vi "pyonpyon3.6.vi"() -> ()   [LabVIEW 2013]
uses:
  impl/pp3_CTL_State.ctl
  impl/pp3_CTL_Trial.ctl
  labolabo2/waveforms/WFTypes.ctl
  impl/pp3_CTL_TrialType.ctl
  <vilib>/Utility/file.llb/Read From Spreadsheet File (string).vi
  labolabo2/array/impl/NullArray_I.vi
  labolabo2/array/impl/ArrayFirst_S.vi
  <vilib>/userdefined/High Color/IMAQdx.ctl
  impl/pp3_CTL_SessionInfo.ctl
  impl/pp3_CTL_StateInfo.ctl
  impl/pp3_CTL_SessionParamDynamic.ctl
  <vilib>/sound2/lvsound2.llb/Sound Output Task ID.ctl
  impl/pp3_CTL_SessionParam.ctl
  impl/pp3c_CTL_DaqStatusVariable.ctl
panel:
  out "Session List Valid":bool=TRUE
  in  "Refresh info":bool
  in  "Session List Hidden":u8[](array[numeric])=[1, 1, 1, 2, 1, 2, 2, 1, 1, 2, 1, 2, 2, 1, 2, 2, 2, 1, 2, 1, 2, 2, 1, 1, 2, 2, 2, 1, 2, 2, 2, 1, 1, 2, 1, 1, 1, 2, 1, 1, 2, 1, 2, 2, 1, 1, 1, 2, 1, 2, 2, 2, 1, 1, 2, 2, 2, 1, 1, 2, 2, 1, 2, 1, 2, 1, 1, 2, 1, 1, 2, 1, 2, 1, 1, 2, 1, 2, 1, 2, 1, 2, 1, 2, 1, 2, 1, 2, 2, 1] min=1 step=1
  out "concatenated string":string="OS Name:                   Microsoft Wi\rOS Version:                6.1.7601 Service Pack 1 Build 7601\rSystem Type:               x64-based PC\rTime Zone:                 (UTC+01:00) Amsterdam, Berli\rTotal Physical Memory:     7,657 MB"
  out "Info VI Revision":string="1300" caption="Rev #"
  out "Info Hostname":string="PCR6985-17"
  out "Session list display":string[][](table)=[["1", "1", "1", "2", "1"], ["2", "2", "1", "1", "2"], ["1", "2", "2", "1", "2"], ["2", "2", "1", "2", "1"], ["2", "2", "1", "1", "2"], ["2", "2", "1", "2", "2"], ["2", "1", "1", "2", "1"], ["1", "1", "2", "1", "1"], ["2", "1", "2", "2", "1"], ["1", "1", "2", "1", "2"], ["2", "2", "1", "1", "2"], ["2", "2", "1", "1", "2"], ["2", "1", "2", "1", "2"], ["1", "1", "2", "1", "1"], ["2", "1", "2", "1", "1"], ["2", "1", "2", "1", "2"], ["1", "2", "1", "2", "1"], ["2", "1", "2", "2", "1"]]
  in  "Trial Types Control":enum32{"Trial Types Control"}(tab)
  out "Trial Types File Path":path=path "E:/Data/SPP.Coulb1/trial types/01_02__FM2k4k_4k2k.pp2tt.tsv"
  in  "Save Trial Types":bool
  in  "Load Trial Types":bool
  out "Trial Types Valid":bool=TRUE
  in  "Trial Types":T1[](array[typedef])=[{"Trial Type Number"=191, "Trial Type"=enum."GO", "Trial Weight"=1, "Shock (mA)"=-1.0, "Duration (ms)"=250.0, "Sound Type"=enum."01 DC", "Stim P1"=1000.0, "Stim P2"=0.0, "Stim P3"=0.0, "Stim P4"=1001.0, "DAQ Amplitude (V)"=0.0}, {"Trial Type Number"=192, "Trial Type"=enum."GO", "Trial Weight"=1, "Shock (mA)"=-1.0, "Duration (ms)"=250.0, "Sound Type"=enum."01 DC", "Stim P1"=1000.0, "Stim P2"=0.0, "Stim P3"=0.0, "Stim P4"=1002.0, "DAQ Amplitude (V)"=0.0}, {"Trial Type Number"=193, "Trial Type"=enum."GO", "Trial Weight"=1, "Shock (mA)"=-1.0, "Duration (ms)"=250.0, "Sound Type"=enum."01 DC", "Stim P1"=1000.0, "Stim P2"=0.0, "Stim P3"=0.0, "Stim P4"=1003.0, "DAQ Amplitude (V)"=0.0}, {"Trial Type Number"=255, "Trial Type"=enum."NOGO", "Trial Weight"=3, "Shock (mA)"=-1.0, "Duration (ms)"=250.0, "Sound Type"=enum."01 DC", "Stim P1"=1000.0, "Stim P2"=0.0, "Stim P3"=0.0, "Stim P4"=0.0, "DAQ Amplitude (V)"=0.0}] {"DAQ Amplitude (V)" min=0.0 max=5.0 format="%_4g"; "Shock (mA)" min=-1.0 max=5.0; "Trial Weight" step=1; "Duration (ms)" min=0.0 max=1.0; "Trial Type Number" min=1 max=256 step=1}
  in  "Session List Control":enum32{"Session List Control"}(tab)
  out "Session List File Path":path
  in  "Load Session List":bool
  in  "Save Session List":bool
  in  "Generate Session List":bool
  in  "Total Trials":i32=90 min=3 max=122 step=1
  in  "Pseudo-Gell. Start":i32=2 min=0 max=3 step=1
  in  "60 trials":bool
  in  "90 trials":bool
  in  "test trials":bool
  in  "Daq config":T4={"Sound AO"="Dev6/ao0", "Shock intesity AO"="Dev6/ao1", "Code_LED DO"="Dev6/port1:2", "Switch DI"="Dev6/port0/line0", "Webcam"="cam9", "Sound AO task"="", "Sound card task"=0, "Shock intensity AO task"="", "Code_LED DO task"="", "Switch DI task"="", "AO <=> Sound card"=FALSE, "Sound card"=0, "sample rate"=100000.0, "Variable shock"=TRUE, "Webcam on"=TRUE, "Waveform memo"={"t0"=timestamp(0 s since 1904-01-01), "dt"=1.0, "Y"=[]}, "First time"=FALSE, "Tone trigger"="PFI1", "Master-9 DO"="Dev6/port0/line5:7", "Master-9 DO task"=""} {"sample rate" min=8000.0; "Sound card task" format="%.0x"}
  out "Image":T7(plugin-control)
  in  "Session param (dynamic)":T8={"Def M shock (uA)"=700.0, "Def F shock (uA)"=140.0}
  in  "stop":bool
  in  "Pause":bool
  out "State info":T9={"Curr  tr"=90, "Curr (ms)"=22027788, "Cum (ms)"=2126369, "Run loop diff"=12, "Tone countdown (ms)"=777777, "Countdown (ms)"=0, "Curr State"=enum."15 Done", "Prev State"=enum."14 Intertrial Interval", "Rw"=FALSE, "Sw"=TRUE, "Tone\nGate"=FALSE, "Punish"=FALSE, "Current DAQ DO Int"=0, "Current Loaded Trial"={"Trial Type Number"=1, "Trial Type"=enum."GO", "Trial Weight"=1, "Shock (mA)"=700.0, "Duration (ms)"=250.0, "Sound Type"=enum."04 FM Sweep", "Stim P1"=2000.0, "Stim P2"=4000.0, "Stim P3"=0.0, "Stim P4"=0.0, "DAQ Amplitude (V)"=1.0}, "Next Trial (for display purposes)"={"Trial Type Number"=1, "Trial Type"=enum."GO", "Trial Weight"=1, "Shock (mA)"=-1.0, "Duration (ms)"=250.0, "Sound Type"=enum."04 FM Sweep", "Stim P1"=2000.0, "Stim P2"=4000.0, "Stim P3"=0.0, "Stim P4"=0.0, "DAQ Amplitude (V)"=1.0}, "Total trials memo"=90, "State start cum memo (ms)"=2111369, "Last dur jump time memo (ms)"=0, "Last dur shock time memo (ms)"=6007, "Tone repeat memo (ms)"=0, "Webcam on"=FALSE, "Webcam recording"=FALSE, "State update flag"=FALSE, "Last loaded shock voltage"=0.35000000000000003, "Vid upd"=enum."6"} {"Current DAQ DO Int" format="%016b"; "Next Trial (for display purposes)"."DAQ Amplitude (V)" min=0.0 max=5.0 format="%_4g"; "Next Trial (for display purposes)"."Shock (mA)" min=-1.0 max=5.0; "Next Trial (for display purposes)"."Trial Weight" step=1; "Next Trial (for display purposes)"."Duration (ms)" min=0.0 max=1.0; "Next Trial (for display purposes)"."Trial Type Number" min=1 max=256 step=1; "Current Loaded Trial"."DAQ Amplitude (V)" min=0.0 max=5.0 format="%_4g"; "Current Loaded Trial"."Shock (mA)" min=-1.0 max=5.0; "Current Loaded Trial"."Trial Weight" step=1; "Current Loaded Trial"."Duration (ms)" min=0.0 max=1.0; "Current Loaded Trial"."Trial Type Number" min=1 max=256 step=1}
  in  "Session parameters":T11={"Log File Directory Root"=path "E:/Data/SPP.Coulb1", "Subject Name"="SPP074", "Tone repeat (ms)"=0, "Habit tr0 (s)"=180, "ITI min\n(s)"=6, "ITI max\n(s)"=16, "Stay \n(s)"=3, "Run"=TRUE, "Jump time\n(s)"=4, "Start trial"=0, "Log File Directory"=path "E:/Data/SPP.Coulb1/SPP074/161224/161555", "Shock \ndur (s)"=6, "Pre click \n(V)"=0.1, "Click\ndel (s)"=1.0, "Reward CR"=FALSE} {"Click\ndel (s)" min=0.0 step=1.0; "Pre click \n(V)" min=0.0 max=1.0 step=1.0; "Shock \ndur (s)" min=0 step=1; "Stay \n(s)" min=0 step=1; "Start trial" step=1; "Jump time\n(s)" min=0 step=1; "Tone repeat (ms)" min=0 max=1000 step=1; "ITI min\n(s)" min=0 step=1; "ITI max\n(s)" min=0 step=1; "Habit tr0 (s)" min=0 step=1}
  out "Runtime Errors":errorcluster
  in  "Refresh":bool
  out "Session info":T12={"Total  Tr"=90, "G Tr"=45, "G Jump"=0, "G Jump%"=0.0, "N Tr"=45, "N Jump"=1, "N Jump%"=2.2222222222222223, "T Tr"=0, "T Jump"=0, "T Jump%"=nan, "M shock dur (ms)"=6003.133333333333, "F shock dur (ms)"=6005.0, "H latency (ms)"=0.0, "F latency (ms)"=3939.0, "T jump latency (ms)"=0.0} {"T Jump%" format="%.3g"; "N Jump%" format="%.3g"; "G Jump%" format="%.3g"}
  # "Pyonpyon Labview  v3.5 \n(2017.3 KT -- opto trig A)"
  # "60 trials:  180-14-24-5\n90 trials:  180-6-16-3"
  # "Code"
  # "Type"
  # "P 1"
  # "P 2"
  # "P 3"
  # "P 4 (opto)"
  # "Weight"
  # "Shock"
  # "Dur (ms)"
  # "DAQ Ampl (V)"
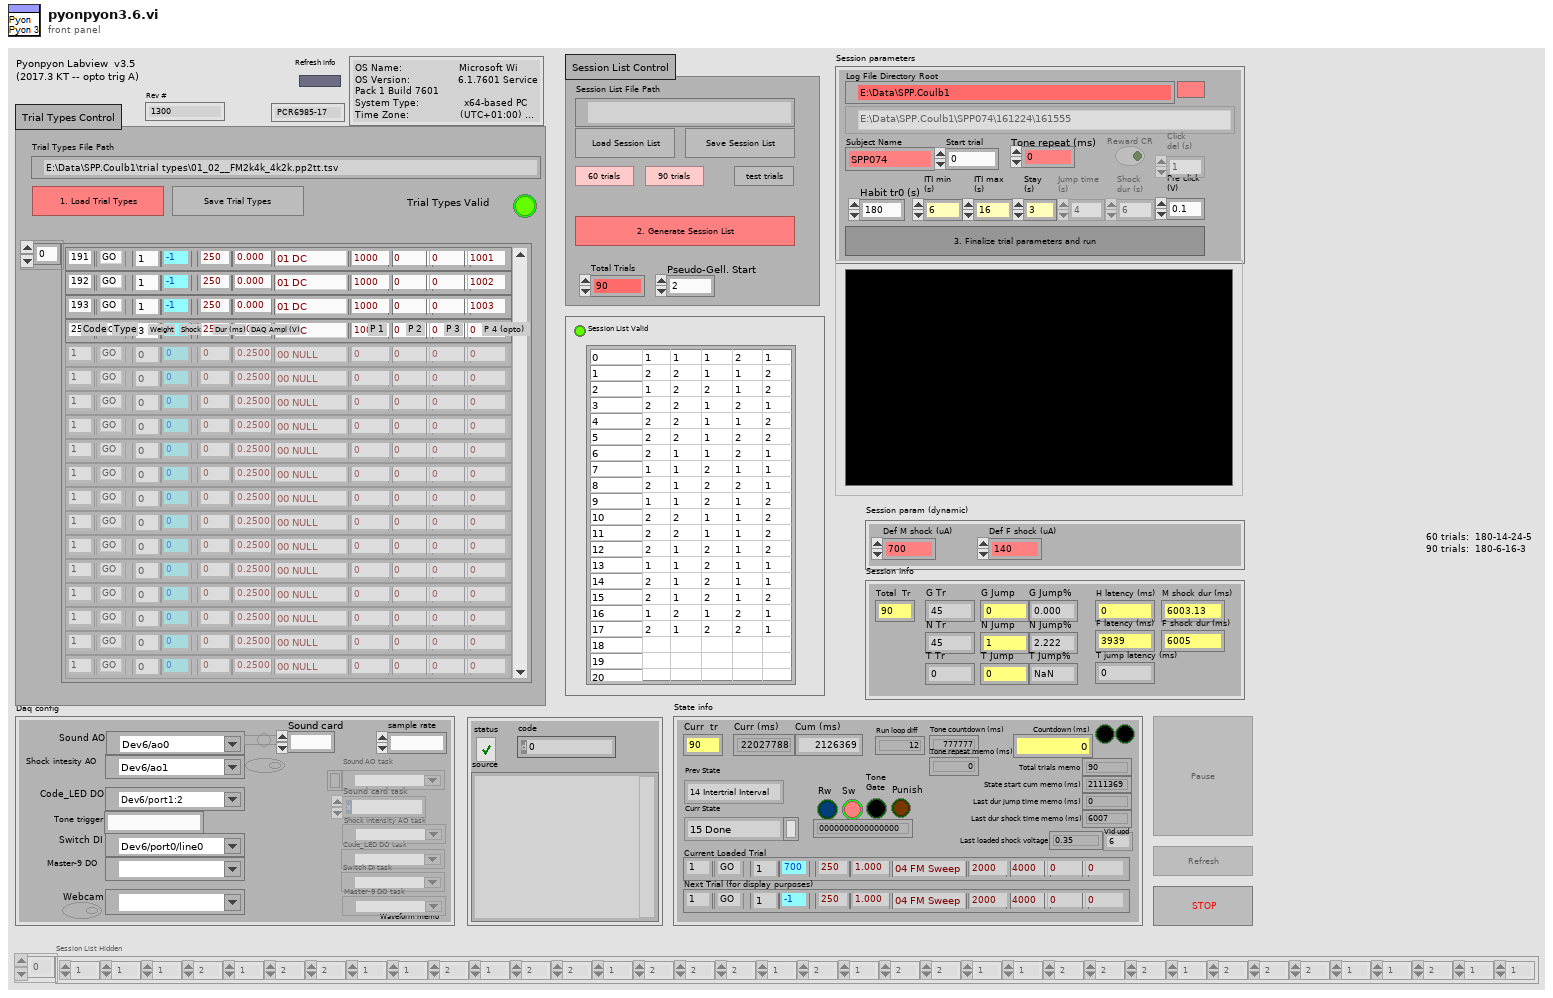
[diagram p1: front panel]
types:
  T1 = typedef "pp3_CTL_Trial.ctl" = cluster{"Trial Type Number":i16, "Trial Type":T2, "Trial Weight":u32, "Shock (mA)":dbl, "Duration (ms)":dbl, "Sound Type":T3, "Stim P1":dbl, "Stim P2":dbl, "Stim P3":dbl, "Stim P4":dbl, "DAQ Amplitude (V)":dbl}
  T2 = typedef "pp3_CTL_TrialType.ctl" = enum16{"OFF", "GO", "NOGO", "TEST"}
  T3 = typedef "WFTypes.ctl" = enum16{"00 NULL", "01 DC", "02 Noise", "03 Pure Tone", "04 FM Sweep"}
  T4 = typedef "pp3c_CTL_DaqStatusVariable.ctl" = cluster{"Sound AO":tag, "Shock intesity AO":tag, "Code_LED DO":tag, "Switch DI":tag, "Webcam":T5, "Sound AO task":refnum<k21>, "Sound card task":T6, "Shock intensity AO task":refnum<k21>, "Code_LED DO task":refnum<k21>, "Switch DI task":refnum<k21>, "AO <=> Sound card":bool, "Sound card":u32, "sample rate":dbl, "Variable shock":bool, "Webcam on":bool, "Waveform memo":waveform(dbl), "First time":bool, "Tone trigger":string, "Master-9 DO":tag, "Master-9 DO task":refnum<k21>}
  T5 = typedef "IMAQdx.ctl" = refnum<k21>
  T6 = typedef "Sound Output Task ID.ctl" = u32
  T7 = typedef "IMAQ Image.ctl" = refnum<image>
  T8 = typedef "pp3_CTL_SessionParamDynamic.ctl" = cluster{"Def M shock (uA)":dbl, "Def F shock (uA)":dbl}
  T9 = typedef "pp3_CTL_StateInfo.ctl" = cluster{"Curr  tr":u16, "Curr (ms)":u32, "Cum (ms)":i64, "Run loop diff":i64, "Tone countdown (ms)":i64, "Countdown (ms)":i64, "Curr State":T10, "Prev State":T10, "Rw":bool, "Sw":bool, "Tone\nGate":bool, "Punish":bool, "Current DAQ DO Int":u16, "Current Loaded Trial":T1, "Next Trial (for display purposes)":T1, "Total trials memo":i64, "State start cum memo (ms)":i64, "Last dur jump time memo (ms)":i64, "Last dur shock time memo (ms)":i64, "Tone repeat memo (ms)":i64, "Webcam on":bool, "Webcam recording":bool, "State update flag":bool, "Last loaded shock voltage":dbl, "Vid upd":enum16{"0", "1", "2", "3", "4", "5", "6", "7", "8", "9"}}
  T10 = typedef "pp3_CTL_State.ctl" = enum8{"0 NULL", "1 Habituation", "2 (Load Trial)", "3 Stay Period", "4 Load Audio/Click Delay", "5 GO Trial", "6 GO Jumped", "7 GO Timeout", "8 NOGO Trial", "9 NOGO Jumped", "10 NOGO Timeout", "11 TEST Trial", "12 TEST Jumped", "13 TEST Timeout", "14 Intertrial Interval", "15 Done"}
  T11 = typedef "pp3_CTL_SessionParam.ctl" = cluster{"Log File Directory Root":path, "Subject Name":string, "Tone repeat (ms)":i32, "Habit tr0 (s)":i32, "ITI min\n(s)":i32, "ITI max\n(s)":i32, "Stay \n(s)":i32, "Run":bool, "Jump time\n(s)":i32, "Start trial":u16, "Log File Directory":path, "Shock \ndur (s)":i32, "Pre click \n(V)":dbl, "Click\ndel (s)":dbl, "Reward CR":bool}
  T12 = typedef "pp3_CTL_SessionInfo.ctl" = cluster{"Total  Tr":u32, "G Tr":u32, "G Jump":u32, "G Jump%":dbl, "N Tr":u32, "N Jump":u32, "N Jump%":dbl, "T Tr":u32, "T Jump":u32, "T Jump%":dbl, "M shock dur (ms)":dbl, "F shock dur (ms)":dbl, "H latency (ms)":dbl, "F latency (ms)":dbl, "T jump latency (ms)":dbl}
  T13 = enum8{"Enabled", "Disabled", "Disabled and Grayed Out"}
  T14 = enum16{"open", "replace", "create", "open or create", "replace or create", "replace or create with confirmation"}
  T15 = typedef "imagedata.ctl" = cluster{"image type":i32, "image depth":i32, "image":u8[], "mask":u8[], "colors":u32[], "Rectangle":cluster{"left":i16, "top":i16, "right":i16, "bottom":i16}}
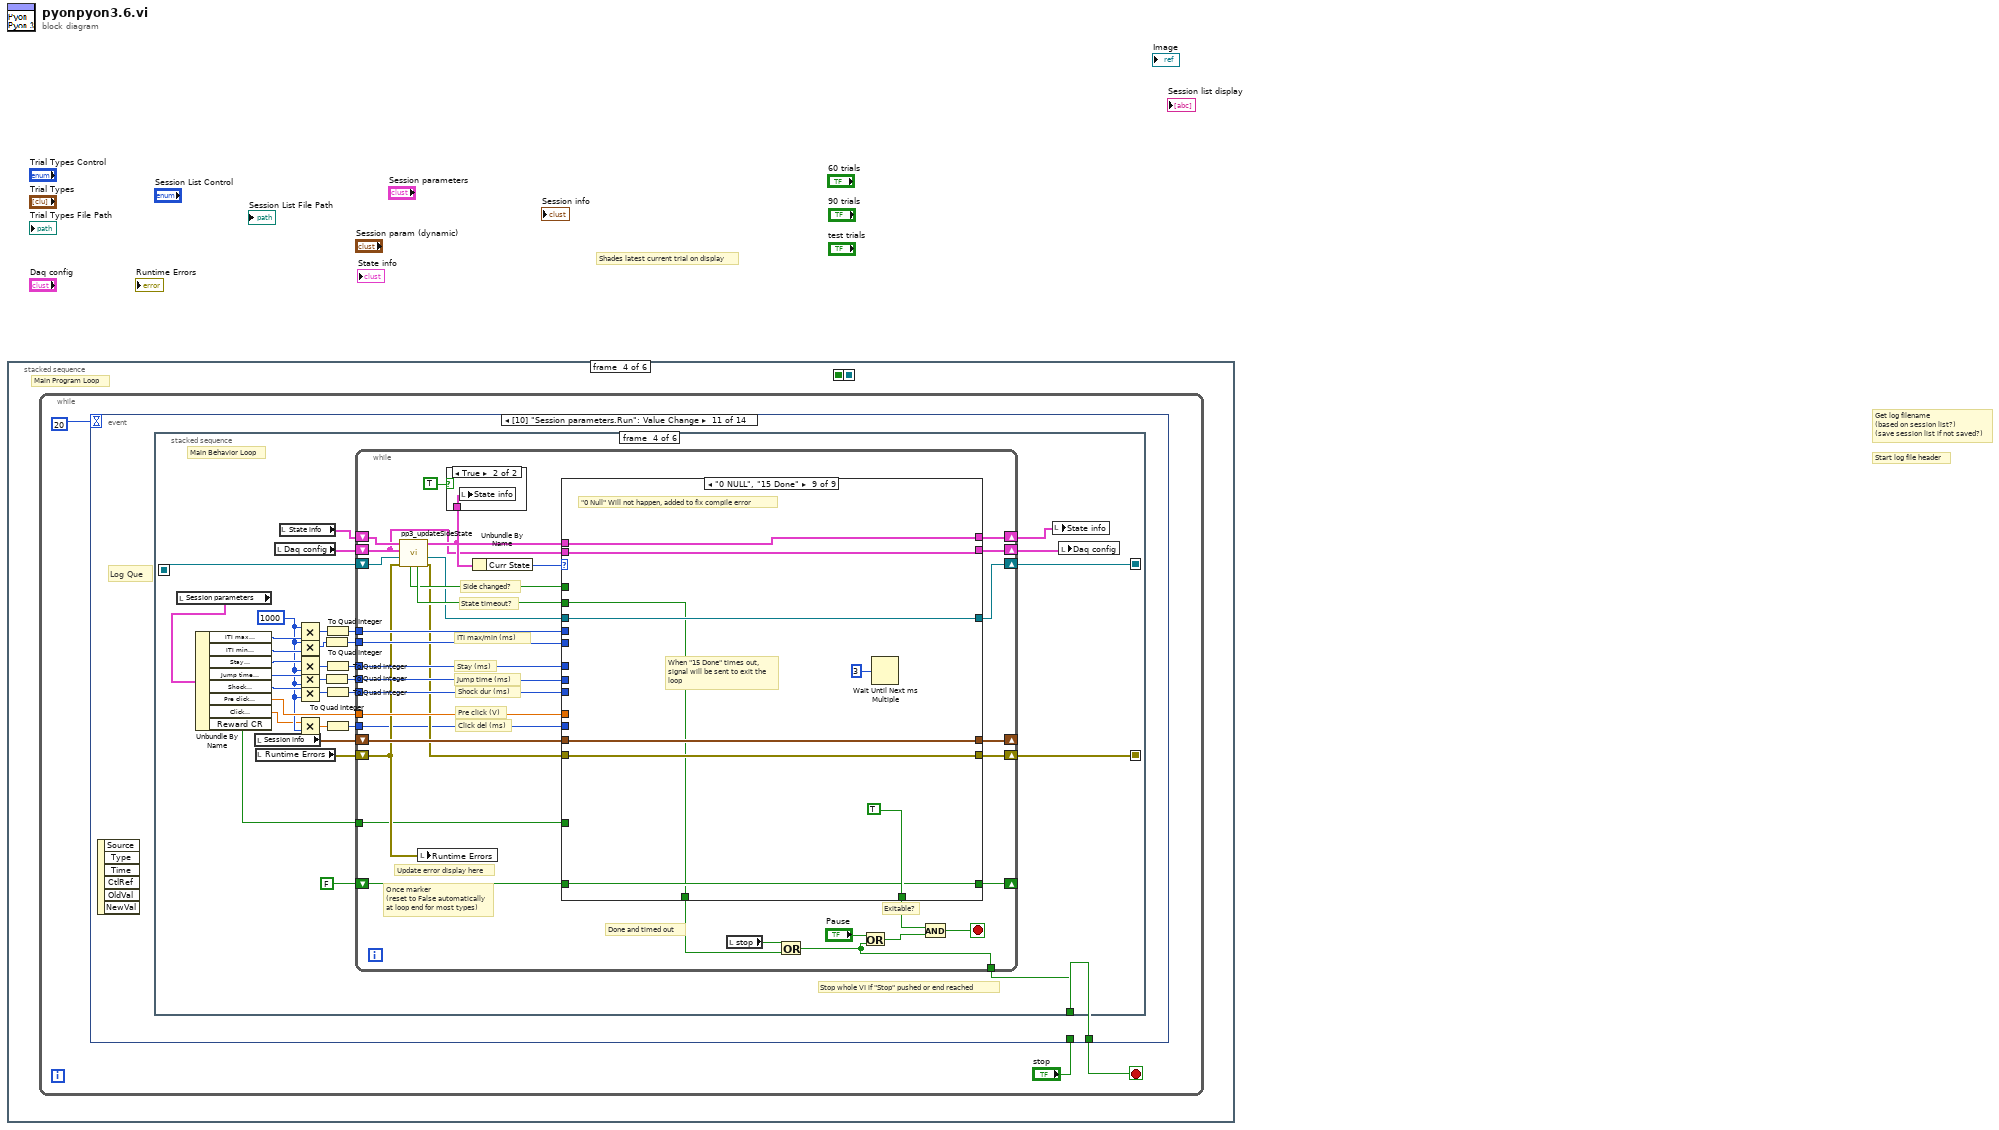
[diagram p0: block diagram]
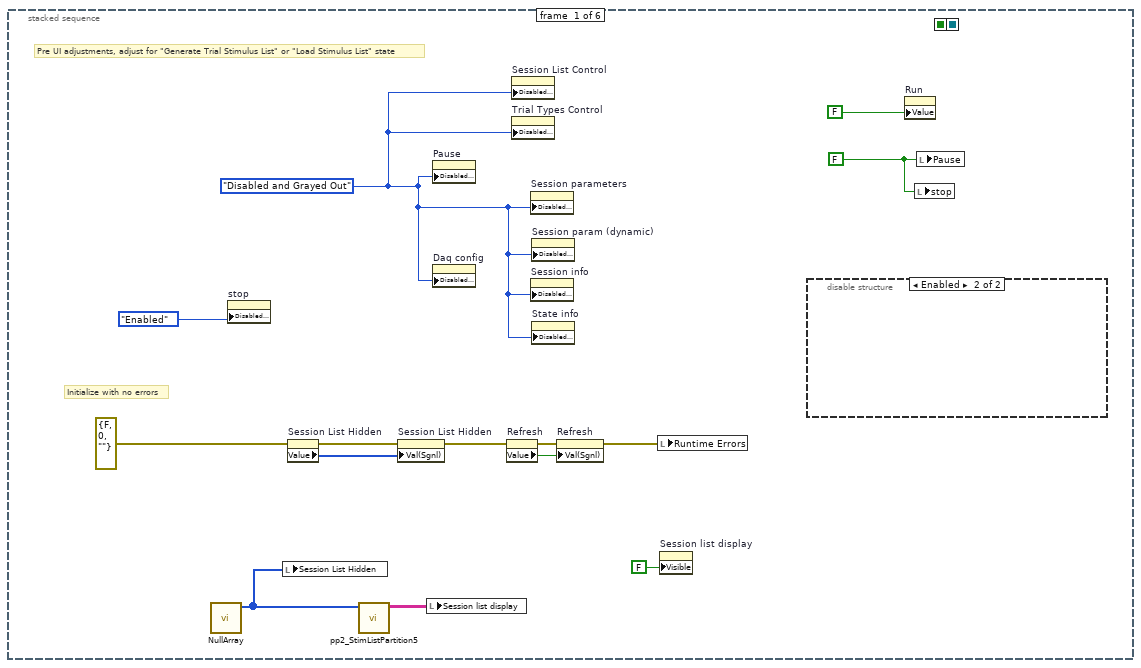
[diagram p2: hidden frame]
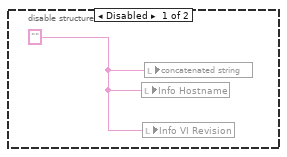
[diagram p3: hidden frame]
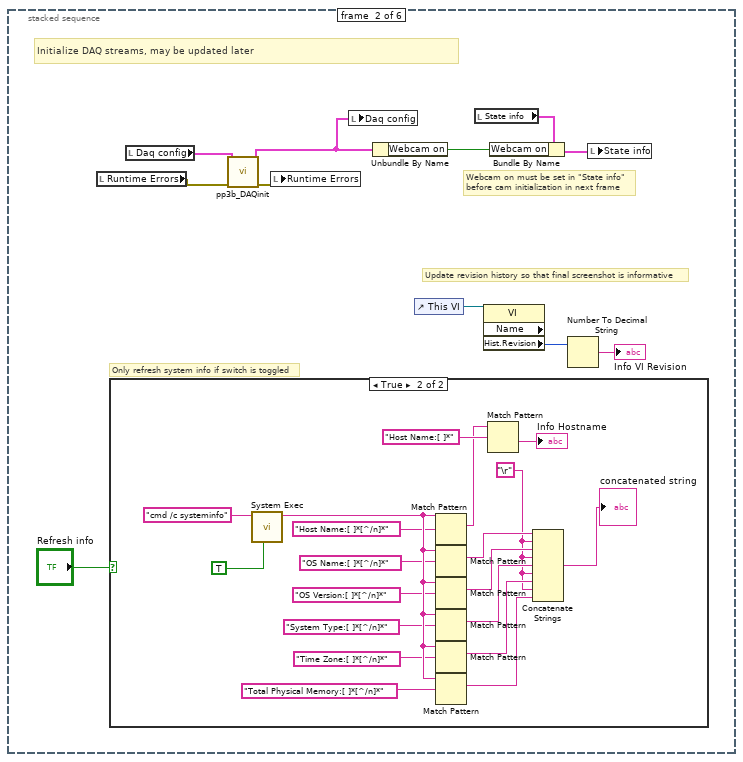
[diagram p4: hidden frame]
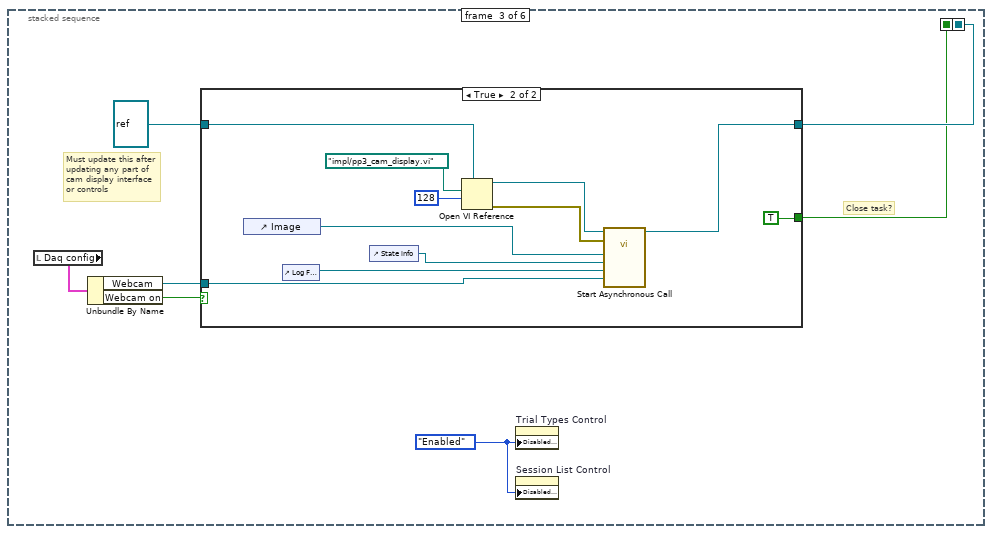
[diagram p6: hidden frame]
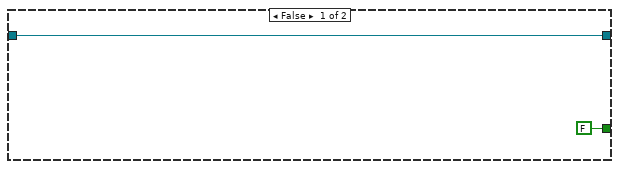
[diagram p7: hidden frame]
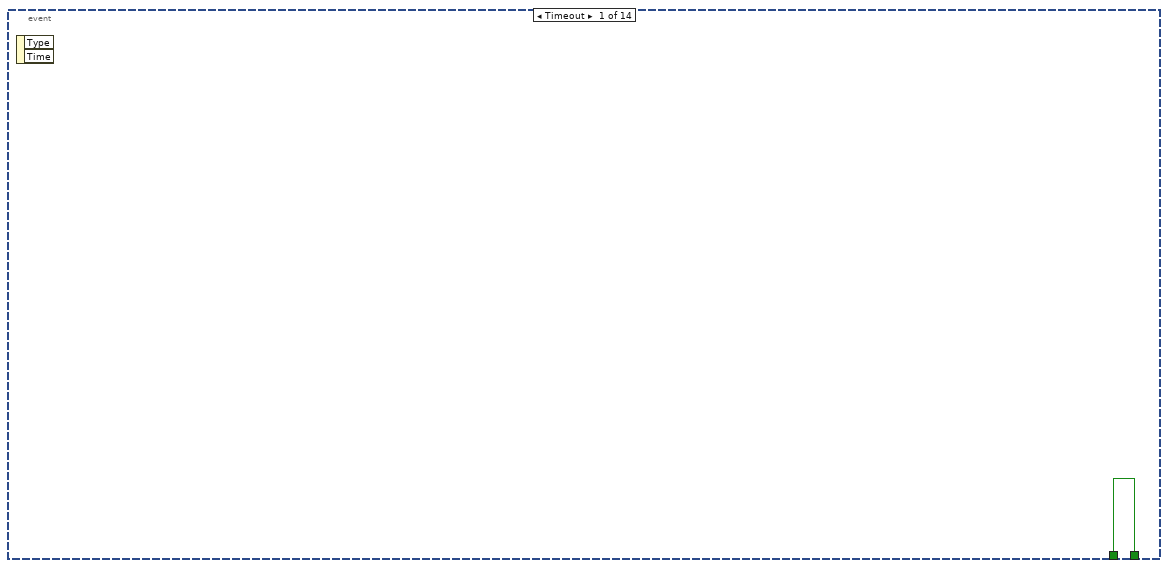
[diagram p8: hidden frame]
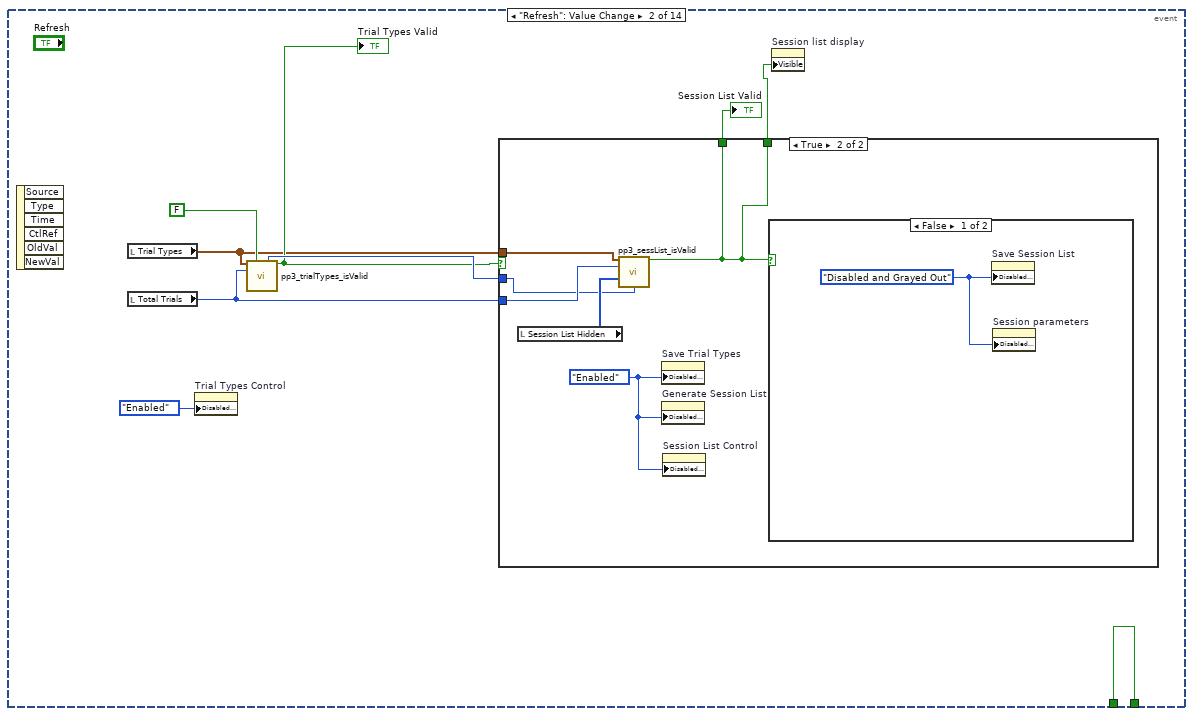
[diagram p9: hidden frame]
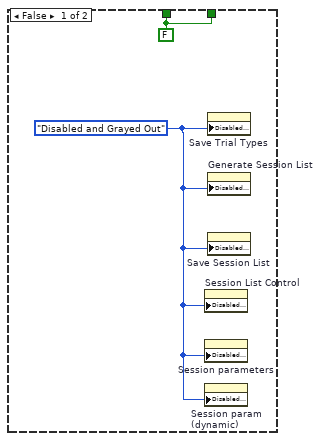
[diagram p10: hidden frame]
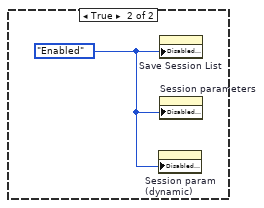
[diagram p11: hidden frame]
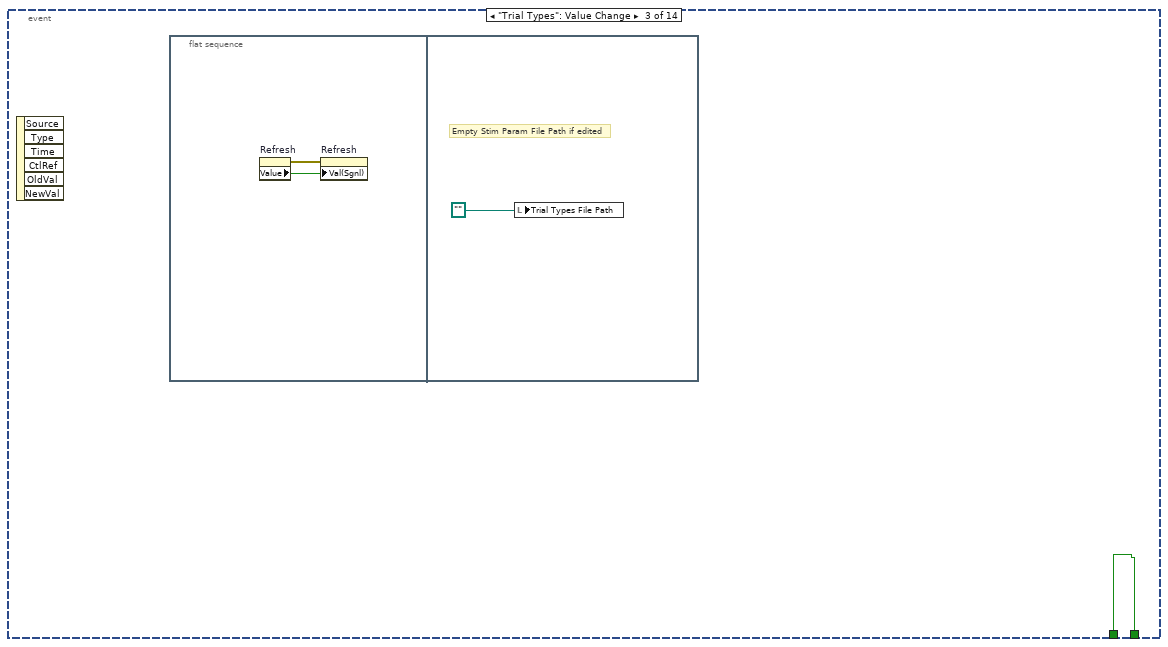
[diagram p12: hidden frame]
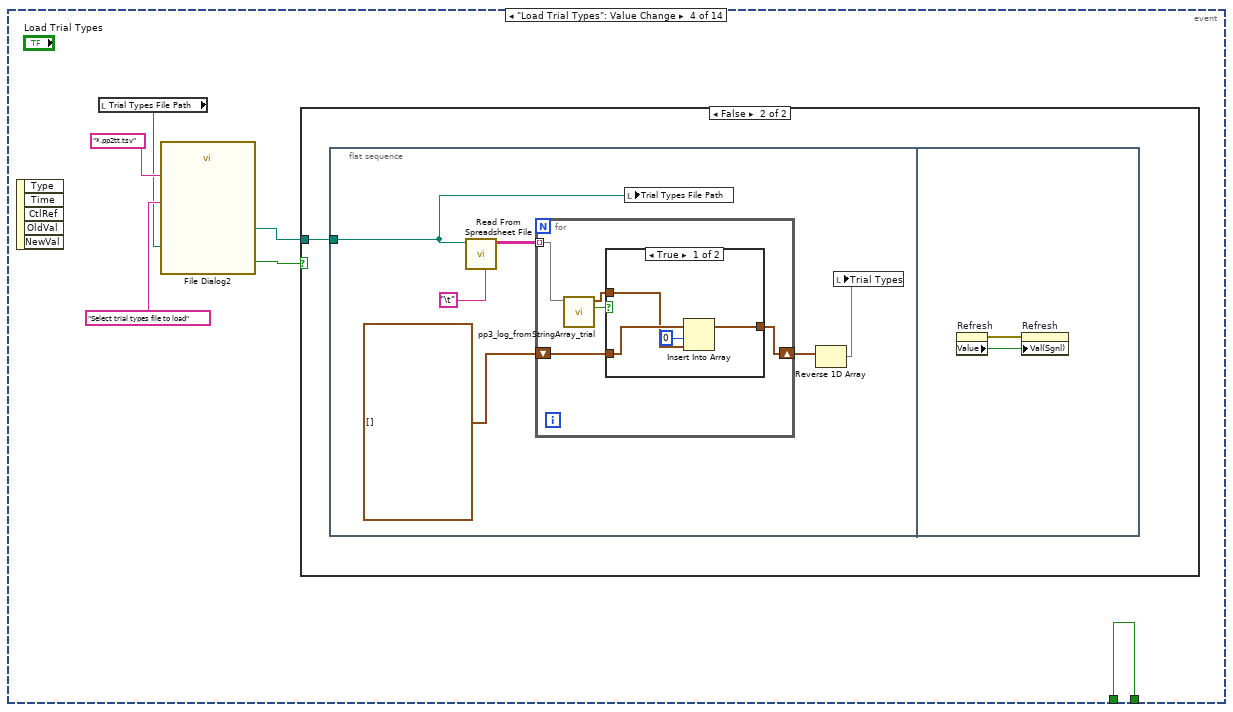
[diagram p13: hidden frame]
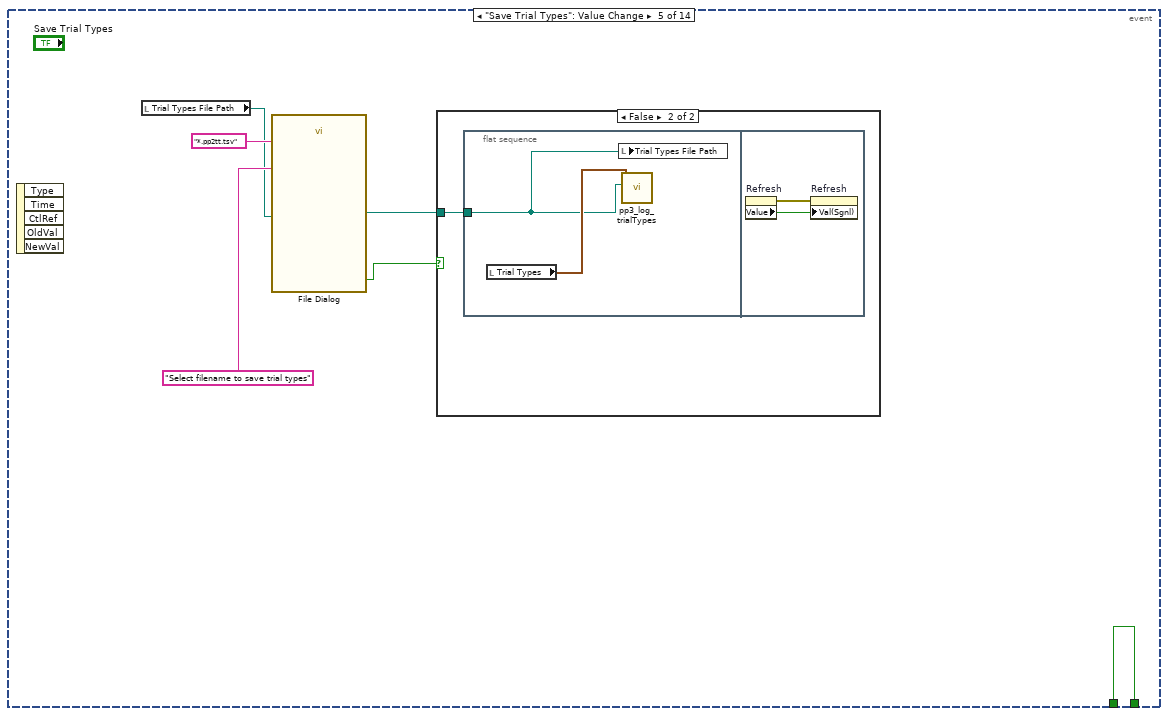
[diagram p16: hidden frame]
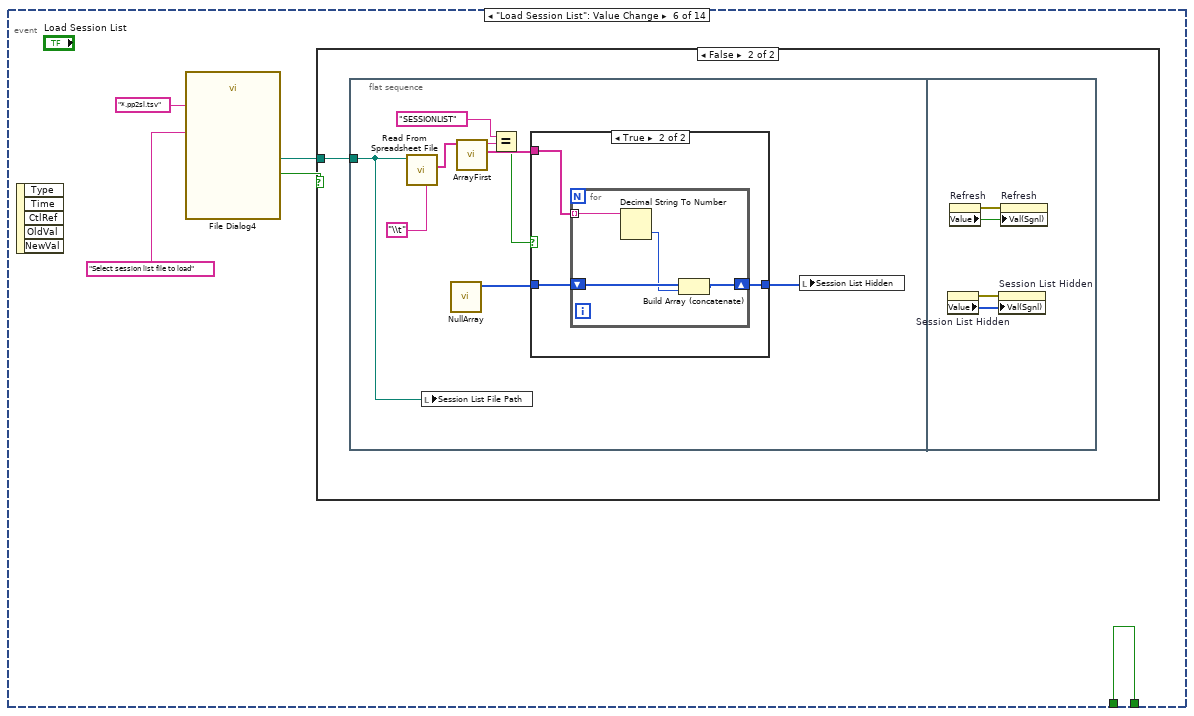
[diagram p18: hidden frame]
diagram:
  # "Shades latest current trial on display"
  # "Start log file header"
  # "Get log filename\n(based on session list?)\n(save session list if not saved?)"
  n1 = stacked-sequence {
    seq-local: [_ _ w49 _ _ _] -> [_ _ _ _ w734 _]
    seq-local: [_ _ w48 _ _ _] -> [_ _ _ _ w731 _]
    frame #0 {
      w14 = FALSE
      w1 = T13."Disabled and Grayed Out" ("Disabled")
      # "Initialize with no errors"
      # "Pre UI adjustments, adjust for \"Generate Trial Stimulus List\" or \"Load Stimulus List\" state"
      n2 = call-poly "NullArray.vi"() -> ("Null Array"=w5:i32[])  [unwired: 11 in]
      n3 = property on="stop" class="Bool (strict)"("DisabledEnum"=T13."Enabled" ("Disabled")) -> ()  [unwired: 2 in, 2 out]
      n4 = local write "Session List Hidden"(w5) -> ()
      n5 = property on="Session List Hidden" class="Arr (strict)"(error in=errorcluster {"status"=FALSE, "code"=0, "source"=""} ("error in (no error)")) -> (error out=w11:errorcluster, "Value"=w10:u8[])  [unwired: 1 in, 1 out]
      n6 = call "pp2_StimListPartition5.vi"("Session List (Hidden variable)"=w5) -> ("Session list display"=w4:string[][])  [unwired: 9 in]
      n7 = property on="Session List Hidden" class="Arr (strict)"(error in=w11, "Val(Sgnl)"=w10) -> (error out=w8:errorcluster)  [unwired: 1 in, 1 out]
      n8 = local write "Session list display"(w4) -> ()
      n9 = property on="Pause" class="Bool (strict)"("DisabledEnum"=w1) -> ()  [unwired: 2 in, 2 out]
      n10 = property on="Daq config" class="Clust (strict)"("DisabledEnum"=w1) -> ()  [unwired: 2 in, 2 out]
      n11 = property on="Refresh" class="Bool (strict)"(error in=w8) -> (error out=w7:errorcluster, "Value"=w9:bool)  [unwired: 1 in, 1 out]
      n12 = property on="Session List Control" class="TabCtl (strict)"("DisabledEnum"=w1) -> ()  [unwired: 2 in, 2 out]
      n13 = property on="Trial Types Control" class="TabCtl (strict)"("DisabledEnum"=w1) -> ()  [unwired: 2 in, 2 out]
      n14 = property on="Session parameters" class="Clust (strict)"("DisabledEnum"=w1) -> ()  [unwired: 2 in, 2 out]
      n15 = property on="Session info" class="Clust (strict)"("DisabledEnum"=w1) -> ()  [unwired: 2 in, 2 out]
      n16 = property on="Session param (dynamic)" class="Clust (strict)"("DisabledEnum"=w1) -> ()  [unwired: 2 in, 2 out]
      n17 = property on="State info" class="Clust (strict)"("DisabledEnum"=w1) -> ()  [unwired: 2 in, 2 out]
      n18 = property on="Refresh" class="Bool (strict)"(error in=w7, "Val(Sgnl)"=w9) -> (error out=w6:errorcluster)  [unwired: 1 in, 1 out]
      n19 = local write "Runtime Errors"(w6) -> ()
      n20 = property on="Session list display" class="Tbl (strict)"("Visible"=FALSE) -> ()  [unwired: 2 in, 2 out]
      n21 = disable-structure shown="Enabled" {
        frame Disabled {
          w15 = "" ("concatenated string")
          n22 = local write "Info Hostname"(w15) -> ()
          n23 = local write "Info VI Revision"(w15) -> ()
          n24 = local write "concatenated string"(w15) -> ()
        }
        frame Enabled {
        }
      }
      n25 = property on="Run" class="Bool (strict)"("Value"=FALSE) -> ()  [unwired: 2 in, 2 out]
      n26 = local write "stop"(w14) -> ()
      n27 = local write "Pause"(w14) -> ()
    }
    frame #1 {
      # "Update revision history so that final screenshot is informative"
      # "Only refresh system info if switch is toggled"
      # "Webcam on must be set in \"State info\"\nbefore cam initialization in next frame"
      # "Initialize DAQ streams, may be updated later"
      n28 = local read "Runtime Errors"() -> (w21:errorcluster)
      n29 = case shown="True" "Refresh info" {
        frame False {
        }
        frame True {
          w35 = "\r"
          n30 = call <vilib>:"System Exec.vi"("run minimized? (F)"=TRUE, "command line"="cmd /c systeminfo") -> ("standard output"=w34:string)  [unwired: 6 in, 3 out]
          n31 = Match Pattern(string=w34, regular expression="Host Name:[ ]*[^/n]*") -> (match substring=w27:string)  [unwired: 1 in, 3 out]
          n32 = Match Pattern(string=w34, regular expression="OS Name:[ ]*[^/n]*") -> (match substring=w41:string)  [unwired: 1 in, 3 out]
          n33 = Match Pattern(string=w34, regular expression="OS Version:[ ]*[^/n]*") -> (match substring=w40:string)  [unwired: 1 in, 3 out]
          n34 = Match Pattern(string=w34, regular expression="System Type:[ ]*[^/n]*") -> (match substring=w39:string)  [unwired: 1 in, 3 out]
          n35 = Match Pattern(string=w34, regular expression="Time Zone:[ ]*[^/n]*") -> (match substring=w38:string)  [unwired: 1 in, 3 out]
          n36 = Match Pattern(string=w34, regular expression="Total Physical Memory:[ ]*[^/n]*") -> (match substring=w37:string)  [unwired: 1 in, 3 out]
          n37 = Match Pattern(string=w27, regular expression="Host Name:[ ]*") -> (after substring=→"Info Hostname":string)  [unwired: 1 in, 3 out]
          n38 = Concatenate Strings(w41, w35, w40, w35, w39, w35, w38, w35, w37) -> (→"concatenated string":string)
        }
      }
      n39 = local read "Daq config"() -> (w26:T4)
      n40 = call "pp3b_DAQinit.vi"("error in (no error)"=w21, "Daq config in"=w26) -> ("error out"=w20:errorcluster, "Daq config out"=w25:T4)  [unwired: 8 in]
      n41 = local write "Runtime Errors"(w20) -> ()
      n42 = local write "Daq config"(w25) -> ()
      n43 = Unbundle By Name(w25) -> ("Webcam on"=w23:bool)
      n44 = control-ref of="This VI"() -> (w19:refnum<vi>)
      n45 = local read "State info"() -> (w24:T9)
      n46 = property class="VI" props=["Name", "Hist.Revision"](reference=w19) -> ("Hist.Revision"=w17:u32)  [unwired: 1 in, 3 out]
      n47 = Bundle By Name(cluster=w24, "Webcam on"=w23) -> (w22:T9)
      n48 = Number To Decimal String(number=w17) -> (decimal integer string=→"Info VI Revision":string)  [unwired: 1 in]
      n49 = local write "State info"(w22) -> ()
    }
    frame #2 {
      w47 = T13."Enabled" ("Disabled")
      # "Close task?"
      # "Must update this after\nupdating any part of\ncam display interface\nor controls"
      n50 = local read "Daq config"() -> (w51:T4)
      n51 = Unbundle By Name(w51) -> ("Webcam"=w52:T5, "Webcam on"=w50:bool)
      n52 = case shown="True" w50 {
        tunnel: w52 -> [_ w56]
        tunnel: [w54 w55] -> w49
        tunnel: refnum<vi> refnum ("type specifier VI Refnum (for type only)") -> [w54 w63]
        tunnel: [FALSE TRUE] -> w48
        frame False {
        }
        frame True {
          n53 = control-ref of="Image"() -> (w59:refnum<vi>)
          n54 = control-ref of="Log File Directory"() -> (w57:refnum<vi>)
          n55 = control-ref of="State info"() -> (w58:refnum<vi>)
          n56 = Open VI Reference(type specifier VI Refnum (for type only)=w63, vi path=path "impl/pp3_cam_display.vi", options=128) -> (vi reference=w60:refnum<vi>, error out=w61:errorcluster)  [unwired: 3 in]
          n57 = call-by-ref "Start Asynchronous Call"(reference=w60, error in=w61, "Camera"=w56, "Log File Directory"=w57, "State info Refnum"=w58, "Image Ctl Refnum"=w59) -> (reference out=w55:refnum<vi>)  [unwired: 8 in, 1 out]
        }
      }
      n58 = property on="Trial Types Control" class="TabCtl (strict)"("DisabledEnum"=w47) -> ()  [unwired: 2 in, 2 out]
      n59 = property on="Session List Control" class="TabCtl (strict)"("DisabledEnum"=w47) -> ()  [unwired: 2 in, 2 out]
    }
    frame #3 {
      # "Main Program Loop"
      n60 = while {
        stop <- w68 stop-if-true
        n61 = event shown="[10] \"Session parameters.Run\": Value Change" {
          selector: _ -> [_ _ _ _ _ _ _ _ _ _ _ _ _ _]
          dyn-events: _ -> [_ _ _ _ _ _ _ _ _ _ _ _ _ _]
          timeout: u32 20 ("milliseconds to wait") -> [_ _ _ _ _ _ _ _ _ _ _ _ _ _]
          tunnel: [w69 w71 w89 w98 w123 w133 w156 w168 w192 w196 w208 w709 w716 w723] -> w68
          tunnel: "stop" -> [w69 w71 w89 w98 w123 w133 w156 w168 w192 w196 _ w709 w716 w723]
          event Timeout {
            n62 = event-data() -> ()  [unwired: 1 in, 2 out]
          }
          event "Refresh": Value Change {
            n63 = event-data() -> ()  [unwired: 1 in, 6 out]
            n64 = local read "Trial Types"() -> (w74:T1[])
            n65 = local read "Total Trials"() -> (w77:i32)
            n66 = property on="Trial Types Control" class="TabCtl (strict)"("DisabledEnum"=T13."Enabled" ("Disabled")) -> ()  [unwired: 2 in, 2 out]
            n67 = call "pp3_trialTypes_isValid.vi"("Trial Types In"=w74, "Throw Error"=FALSE, "Total Trials"=w77) -> ("Trial Replication Factor"=w78:i32, "Paradigm Valid?"=w75:bool)  [unwired: 7 in, 4 out]
            "Trial Types Valid" <- w75
            n68 = case shown="True" w75 {
              tunnel: w78 -> [_ w83]
              tunnel: w77 -> [_ w86]
              tunnel: w74 -> [_ w85]
              tunnel: [w79 w81] -> w73
              tunnel: [w79 w81] -> w70
              frame False {
                w79 = FALSE ("Session List Valid?")
                w80 = T13."Disabled and Grayed Out" ("Disabled")
                n69 = property on="Session List Control" class="TabCtl (strict)"("DisabledEnum"=w80) -> ()  [unwired: 2 in, 2 out]
                n70 = property on="Session parameters" class="Clust (strict)"("DisabledEnum"=w80) -> ()  [unwired: 2 in, 2 out]
                n71 = property on="Session param (dynamic)" class="Clust (strict)"("DisabledEnum"=w80) -> ()  [unwired: 2 in, 2 out]
                n72 = property on="Save Trial Types" class="Bool"("DisabledEnum"=w80) -> ()  [unwired: 2 in, 2 out]
                n73 = property on="Generate Session List" class="Bool"("DisabledEnum"=w80) -> ()  [unwired: 2 in, 2 out]
                n74 = property on="Save Session List" class="Bool"("DisabledEnum"=w80) -> ()  [unwired: 2 in, 2 out]
              }
              frame True {
                w82 = T13."Enabled" ("Disabled")
                n75 = local read "Session List Hidden"() -> (w84:u8[])
                n76 = call "pp3_sessList_isValid.vi"("Trial Types In"=w85, "Total Trials"=w86, "Session List"=w84, "Trial Replication Factor"=w83) -> ("Session List Valid?"=w81:bool)  [unwired: 11 in]
                n77 = property on="Save Trial Types" class="Bool"("DisabledEnum"=w82) -> ()  [unwired: 2 in, 2 out]
                n78 = property on="Generate Session List" class="Bool"("DisabledEnum"=w82) -> ()  [unwired: 2 in, 2 out]
                n79 = property on="Session List Control" class="TabCtl (strict)"("DisabledEnum"=w82) -> ()  [unwired: 2 in, 2 out]
                n80 = case shown="False" w81 {
                  frame False {
                    w87 = T13."Disabled and Grayed Out" ("Disabled")
                    n81 = property on="Save Session List" class="Bool"("DisabledEnum"=w87) -> ()  [unwired: 2 in, 2 out]
                    n82 = property on="Session parameters" class="Clust (strict)"("DisabledEnum"=w87) -> ()  [unwired: 2 in, 2 out]
                  }
                  frame True {
                    w88 = T13."Enabled" ("Disabled")
                    n83 = property on="Session param (dynamic)" class="Clust (strict)"("DisabledEnum"=w88) -> ()  [unwired: 2 in, 2 out]
                    n84 = property on="Save Session List" class="Bool"("DisabledEnum"=w88) -> ()  [unwired: 2 in, 2 out]
                    n85 = property on="Session parameters" class="Clust (strict)"("DisabledEnum"=w88) -> ()  [unwired: 2 in, 2 out]
                  }
                }
              }
            }
            "Session List Valid" <- w73
            n86 = property on="Session list display" class="Tbl (strict)"("Visible"=w70) -> ()  [unwired: 2 in, 2 out]
          }
          event "Trial Types": Value Change {
            n87 = event-data() -> ()  [unwired: 1 in, 6 out]
            n88 = flat-sequence {
              frame #0 {
                n89 = property on="Refresh" class="Bool (strict)"() -> (error out=w91:errorcluster, "Value"=w90:bool)  [unwired: 2 in, 1 out]
                n90 = property on="Refresh" class="Bool (strict)"(error in=w91, "Val(Sgnl)"=w90) -> ()  [unwired: 1 in, 2 out]
              }
              frame #1 {
                # "Empty Stim Param File Path if edited"
                n91 = local write "Trial Types File Path"(path "") -> ()
              }
            }
          }
          event "Load Trial Types": Value Change {
            n92 = event-data() -> ()  [unwired: 1 in, 5 out]
            n93 = local read "Trial Types File Path"() -> (w93:path)
            n94 = call "File Dialog2"("start path"=w93, "prompt"="Select trial types file to load", "pattern (all files)"="*.pp2tt.tsv") -> ("selected path"=w95:path, "cancelled"=w94:bool)  [unwired: 9 in, 2 out]
            n95 = case shown="False" w94 {
              tunnel: w95 -> [_ w99]
              frame True {
              }
              frame False {
                n96 = flat-sequence {
                  tunnel: w99 -> [w101]
                  frame #0 {
                    n97 = call-poly <vilib>:"Read From Spreadsheet File.vi"("delimiter (\\t)"="\t" ("delimiter (\\t)"), "file path (dialog if empty)"=w101) -> ("all rows"=w105:string[][])  [unwired: 5 in, 4 out]
                    n98 = for {
                      tunnel: w105 -> [w109] mode=indexing
                      shift-right: [w107] -> w103
                      shift-left: T1[] [] -> [w108]
                      n99 = call "pp3_log_fromStringArray_trial.vi"("Input string array"=w109) -> ("Was TRIAL?"=w106:bool, "Trial in"=w110:T1)  [unwired: 7 in]
                      n100 = case shown="True" w106 {
                        tunnel: w110 -> [w113 _]
                        tunnel: w108 -> [w114 w115]
                        tunnel: [w111 w115] -> w107
                        frame True {
                          n101 = Insert Into Array(array=w114, index=0, new element=w113) -> (w111:T1[])
                        }
                        frame False {
                        }
                      }
                    }
                    n102 = local write "Trial Types File Path"(w101) -> ()
                    n103 = Reverse 1D Array(array=w103) -> (reversed array=w102:T1[])
                    n104 = local write "Trial Types"(w102) -> ()
                  }
                  frame #1 {
                    n105 = property on="Refresh" class="Bool (strict)"() -> (error out=w117:errorcluster, "Value"=w116:bool)  [unwired: 2 in, 1 out]
                    n106 = property on="Refresh" class="Bool (strict)"(error in=w117, "Val(Sgnl)"=w116) -> ()  [unwired: 1 in, 2 out]
                  }
                }
              }
            }
          }
          event "Save Trial Types": Value Change {
            n107 = event-data() -> ()  [unwired: 1 in, 5 out]
            n108 = local read "Trial Types File Path"() -> (w119:path)
            n109 = call "File Dialog"("start path"=w119, "prompt"="Select filename to save trial types", "pattern (all files)"="*.pp2tt.tsv") -> ("selected path"=w120:path, "cancelled"=w118:bool)  [unwired: 9 in, 2 out]
            n110 = case shown="False" w118 {
              tunnel: w120 -> [_ w124]
              frame True {
              }
              frame False {
                n111 = flat-sequence {
                  tunnel: w124 -> [w125]
                  frame #0 {
                    n112 = local read "Trial Types"() -> (w126:T1[])
                    n113 = local write "Trial Types File Path"(w125) -> ()
                    n114 = call "pp3_log_trialTypes.vi"("Trial Types File Path"=w125, "Trial Types"=w126) -> ()  [unwired: 10 in]
                  }
                  frame #1 {
                    n115 = property on="Refresh" class="Bool (strict)"() -> (error out=w127:errorcluster, "Value"=w128:bool)  [unwired: 2 in, 1 out]
                    n116 = property on="Refresh" class="Bool (strict)"(error in=w127, "Val(Sgnl)"=w128) -> ()  [unwired: 1 in, 2 out]
                  }
                }
              }
            }
          }
          event "Load Session List": Value Change {
            n117 = event-data() -> ()  [unwired: 1 in, 5 out]
            n118 = call "File Dialog4"("prompt"="Select session list file to load", "pattern (all files)"="*.pp2sl.tsv") -> ("selected path"=w130:path, "cancelled"=w129:bool)  [unwired: 10 in, 2 out]
            n119 = case shown="False" w129 {
              tunnel: w130 -> [_ w134]
              frame True {
              }
              frame False {
                n120 = flat-sequence {
                  tunnel: w134 -> [w138]
                  frame #0 {
                    n121 = call-poly <vilib>:"Read From Spreadsheet File.vi"("delimiter (\\t)"="\\t" ("delimiter (\\t)"), "file path (dialog if empty)"=w138) -> ("first row"=w142:string[])  [unwired: 5 in, 4 out]
                    n122 = local write "Session List File Path"(w138) -> ()
                    n123 = call-poly "NullArray.vi"() -> ("Null Array"=w135:i32[])  [unwired: 11 in]
                    n124 = call-poly "ArrayFirst.vi"("1D Array In"=w142) -> ("Rest of Array"=w139:string[], "First Element"=w141:string)  [unwired: 9 in]
                    n125 = Equal?(x="SESSIONLIST", y=w141) -> (x = y?=w137:bool)
                    n126 = case shown="True" w137 {
                      tunnel: w139 -> [_ w147]
                      tunnel: [w144 w146] -> w136
                      tunnel: w135 -> [w144 w145]
                      frame False {
                      }
                      frame True {
                        n127 = for {
                          shift-right: [w151] -> w146
                          shift-left: w145 -> [w150]
                          tunnel: w147 -> [w149] mode=indexing
                          n128 = Decimal String To Number(string=w149) -> (number=w148:i32)  [unwired: 2 in, 1 out]
                          n129 = Build Array (concatenate)(w150, w148) -> (w151:i32[])
                        }
                      }
                    }
                    n130 = local write "Session List Hidden"(w136) -> ()
                  }
                  frame #1 {
                    n131 = property on="Session List Hidden" class="Arr (strict)"() -> (error out=w152:errorcluster, "Value"=w153:u8[])  [unwired: 2 in, 1 out]
                    n132 = property on="Refresh" class="Bool (strict)"() -> (error out=w155:errorcluster, "Value"=w154:bool)  [unwired: 2 in, 1 out]
                    n133 = property on="Session List Hidden" class="Arr (strict)"(error in=w152, "Val(Sgnl)"=w153) -> ()  [unwired: 1 in, 2 out]
                    n134 = property on="Refresh" class="Bool (strict)"(error in=w155, "Val(Sgnl)"=w154) -> ()  [unwired: 1 in, 2 out]
                  }
                }
              }
            }
          }
          event "Save Session List": Value Change {
            n135 = event-data() -> ()  [unwired: 1 in, 5 out]
            n136 = flat-sequence {
              frame #0 {
                n137 = call "File Dialog3"("prompt"="Select filename to save session list", "pattern (all files)"="*.pp2sl.tsv") -> ("selected path"=w160:path, "cancelled"=w159:bool)  [unwired: 10 in, 2 out]
                n138 = case shown="False" w159 {
                  tunnel: w160 -> [_ w163]
                  frame True {
                  }
                  frame False {
                    n139 = local read "Session List Hidden"() -> (w165:u8[])
                    n140 = call "pp2_log_toString_sessionList.vi"("Session List in"=w165) -> ("spreadsheet string"=w164:string)  [unwired: 10 in]
                    n141 = Write to Text File(file (use dialog)=w163, text=w164) -> (refnum out=w161:refnum<file>, error out=w162:errorcluster)  [unwired: 2 in, 1 out]
                    n142 = Close File(refnum=w161, error in=w162) -> ()  [unwired: 2 out]
                    n143 = local write "Session List File Path"(w163) -> ()
                  }
                }
              }
              frame #1 {
                n144 = property on="Refresh" class="Bool (strict)"() -> (error out=w167:errorcluster, "Value"=w166:bool)  [unwired: 2 in, 1 out]
                n145 = property on="Refresh" class="Bool (strict)"(error in=w167, "Val(Sgnl)"=w166) -> ()  [unwired: 1 in, 2 out]
              }
            }
          }
          event "Generate Session List": Value Change {
            n146 = event-data() -> ()  [unwired: 1 in, 5 out]
            n147 = flat-sequence {
              frame #0 {
                # "Empty file name if generating list"
                n148 = local read "Trial Types"() -> (w175:T1[])
                n149 = local read "Total Trials"() -> (w169:i32)
                n150 = Array Size(array=w175) -> (size(s)=w174:i32)
                n151 = Equal?(x=w174, y=1) -> (x = y?=w172:bool)
                n152 = case shown="False" w172 {
                  tunnel: w175 -> [w181 w184]
                  tunnel: [w176 w183] -> w170
                  tunnel: w169 -> [w177 w182]
                  frame True {
                    # "If only one trial type, just\nrepetitions of that trial in a row"
                    n153 = Index Array(array=w181, index=0) -> (element=w179:T1)
                    n154 = Unbundle By Name(w179) -> ("Trial Type Number"=w178:i16)
                    n155 = Initialize Array(w178, w177) -> (w176:i16[])
                  }
                  frame False {
                    n156 = call "pp3_sessList_createPseudoGellerman.vi"("Start Num"="Pseudo-Gell. Start", "Total Trials"=w182, "Trial Types"=w184) -> ("Session List (Cannot Edit)"=w183:i32[])  [unwired: 7 in, 1 out]
                  }
                }
                n157 = local write "Session List File Path"(path "") -> ()
                n158 = local write "Session List Hidden"(w170) -> ()
              }
              frame #1 {
                n159 = property on="Session List Hidden" class="Arr (strict)"() -> (error out=w187:errorcluster, "Value"=w186:u8[])  [unwired: 2 in, 1 out]
                n160 = property on="Session list display" class="Tbl (strict)"() -> (error out=w189:errorcluster, "Value"=w188:string[][])  [unwired: 2 in, 1 out]
                n161 = property on="Refresh" class="Bool (strict)"() -> (error out=w191:errorcluster, "Value"=w190:bool)  [unwired: 2 in, 1 out]
                n162 = property on="Session list display" class="Tbl (strict)"(error in=w189, "Val(Sgnl)"=w188) -> ()  [unwired: 1 in, 2 out]
                n163 = property on="Refresh" class="Bool (strict)"(error in=w191, "Val(Sgnl)"=w190) -> ()  [unwired: 1 in, 2 out]
                n164 = property on="Session List Hidden" class="Arr (strict)"(error in=w187, "Val(Sgnl)"=w186) -> ()  [unwired: 1 in, 2 out]
              }
            }
          }
          event "Total Trials": Value Change {
            n165 = event-data() -> ()  [unwired: 1 in, 6 out]
            n166 = flat-sequence {
              tunnel: "Total Trials" -> [_]
              frame #0 {
              }
              frame #1 {
                n167 = property on="Refresh" class="Bool (strict)"() -> (error out=w194:errorcluster, "Value"=w195:bool)  [unwired: 2 in, 1 out]
                n168 = property on="Refresh" class="Bool (strict)"(error in=w194, "Val(Sgnl)"=w195) -> ()  [unwired: 1 in, 2 out]
              }
            }
          }
          event "Session List Hidden": Value Change {
            # "Run thru all rows/columns and paint white"
            # "Refresh row headers on left"
            # "Refresh session list grid display"
            n169 = event-data() -> ()  [unwired: 1 in, 6 out]
            n170 = for {
              N: 24 -> [_]
              tunnel: [w201] -> w197 mode=indexing
              i -> [w202]
              # "rows"
              n171 = for {
                N: 5 -> [_]
                tunnel: w202 -> [w207]
                i -> [w206]
                # "columns"
                # "Blank white\ncolor"
                n172 = Bundle(w207, w206) -> (w205:cluster{i32, i32})  [unwired: 1 in]
                n173 = property on="Session list display" class="Tbl (strict)"("Active Cell"=w205, "Cell BG Color"=u32 16448250) -> ()  [unwired: 2 in, 2 out]
              }
              n174 = Number To Decimal String(number=w202) -> (decimal integer string=w201:string)  [unwired: 1 in]
            }
            n175 = call "pp2_StimListPartition5.vi"("Session List (Hidden variable)"="Session List Hidden") -> ("Session list display"=w199:string[][])  [unwired: 9 in]
            n176 = local write "Session list display"(w199) -> ()
            n177 = property on="Session list display" class="Tbl (strict)"("Row Headers[]"=w197) -> ()  [unwired: 2 in, 2 out]
          }
          event Value Change {
            # "Log Que"
            n178 = event-data() -> ()  [unwired: 1 in, 6 out]
            n179 = stacked-sequence {
              seq-local: [_ _ w281 _ _ _] -> [_ _ _ w326 _ _]
              seq-local: [_ _ _ w336 _ _] -> [_ _ _ _ w696 _]
              seq-local: [_ _ _ w324 _ _] -> [_ _ _ _ w695 _]
              tunnel: [_ _ _ w325 _ _] -> w208
              frame #0 {
                w209 = T13."Disabled" ("Disabled")
                w210 = T13."Disabled and Grayed Out" ("Disabled")
                # "Confirm if starting with nonzero trial"
                # "GUI Adjustments (pre)"
                n180 = local read "Session parameters"() -> (w211:T11)
                n181 = flat-sequence {
                  tunnel: w210 -> [w215]
                  frame #0 {
                    n182 = property on="Session List Control" class="TabCtl (strict)"("DisabledEnum"=w215) -> ()  [unwired: 2 in, 2 out]
                  }
                  frame #1 {
                    n183 = property on="Session list display" class="Tbl (strict)"("DisabledEnum"=T13."Disabled" ("Disabled")) -> ()  [unwired: 2 in, 2 out]
                  }
                }
                n184 = Unbundle By Name(w211) -> ("Start trial"=w212:u16)
                n185 = property on="Trial Types Control" class="TabCtl (strict)"("DisabledEnum"=w210) -> ()  [unwired: 2 in, 2 out]
                n186 = property on="Session parameters" class="Clust (strict)"("DisabledEnum"=w210) -> ()  [unwired: 2 in, 2 out]
                n187 = Not Equal To 0?(x=w212) -> (x != 0?=w213:bool)
                n188 = case shown="True" w213 {
                  tunnel: w212 -> [_ w220]
                  tunnel: w211 -> [_ w217]
                  frame False {
                  }
                  frame True {
                    n189 = Number To Decimal String(number=w220) -> (decimal integer string=w221:string)  [unwired: 1 in]
                    n190 = Concatenate Strings("Really start with nonzero trial?: " ("message"), w221) -> (w219:string)
                    n191 = Two Button Dialog(message=w219, 1:"No, start from zero" ("F button name (\"Cancel\")"), 2:"Yes" ("T button name (\"OK\")")) -> (T button?=w218:bool)
                    n192 = case shown="False" w218 {
                      tunnel: w217 -> [w227 _]
                      frame False {
                        n193 = Bundle By Name(cluster=w227, "Start trial"=u16 0) -> (w225:T11)
                        n194 = local write "Session parameters"(w225) -> ()
                      }
                      frame True {
                        # "Just proceed"
                      }
                    }
                  }
                }
                n195 = disable-structure shown="Disabled" {
                  frame Disabled {
                    n196 = property on="Pause" class="Bool (strict)"("DisabledEnum"=T13."Enabled" ("Disabled")) -> ()  [unwired: 2 in, 2 out]
                  }
                  frame Enabled {
                  }
                }
                n197 = property on="State info" class="Clust (strict)"("DisabledEnum"=w209) -> ()  [unwired: 2 in, 2 out]
                n198 = property on="Session info" class="Clust (strict)"("DisabledEnum"=w209) -> ()  [unwired: 2 in, 2 out]
              }
              frame #1 {
                # "ToDo... go through\nsequence for starting\nat trial !=0 for new\nlog, when state info is not\ninitialized yet!"
                # "If webcam is on, start recording"
                # "Reset trial to zero if exceeded total"
                # "If starting from trial zero, clear and habituate, if not, directly to load trial"
                # "Pre-behavior state and statistics adjustments"
                n199 = local read "Session parameters"() -> (w246:T11)
                n200 = Unbundle By Name(w246) -> ("Start trial"=w241:u16, "Habit tr0 (s)"=w229:i32, "Tone repeat (ms)"=w237:i32, "Reward CR"=w228:bool)
                n201 = local read "Session List Hidden"() -> (w239:u8[])
                n202 = Array Size(array=w239) -> (size(s)=w238:i32)
                n203 = Greater Than 0?(x=w229) -> (x > 0?=w232:bool)
                n204 = Greater Or Equal?(x=w241, y=w238) -> (x >= y?=w242:bool)
                n205 = case shown="True" w242 {
                  tunnel: w241 -> [w260 _]
                  tunnel: [w260 u16 0 ("Curr  tr")] -> w240
                  frame False {
                  }
                  frame True {
                  }
                }
                n206 = Equal To 0?(x=w240) -> (x = 0?=w230:bool)
                n207 = And(x=w230, y=w232) -> (x .and. y?=w231:bool)
                n208 = local read "State info"() -> (w236:T9)
                n209 = Unbundle By Name(w236) -> ("Webcam on"=w235:bool)
                n210 = Bundle By Name(cluster=w236, "Curr  tr"=w240, "Curr State"=pp3_CTL_State."1 Habituation", "Prev State"=pp3_CTL_State."0 NULL", "Total trials memo"=w238, "Tone repeat memo (ms)"=w237, "Webcam recording"=w235) -> (w243:T9)
                n211 = case shown="True" w230 {
                  tunnel: w243 -> [w262 w269]
                  tunnel: w229 -> [_ _]
                  tunnel: [w262 w263] -> w234
                  frame False {
                  }
                  frame True {
                    # "Reset time and info only\nif for 0th trial????!!!"
                    n212 = Tick Count (ms)() -> (millisecond timer value=w268:u32)
                    n213 = To Quad Integer(1:w268) -> (0:w267:i64)
                    n214 = Bundle By Name(cluster=w269, "Curr (ms)"=w267, "Cum (ms)"=i64 0) -> (w263:T9)
                    n215 = local read "Session info"() -> (w264:T12)
                    n216 = call "pp2_updateSessionInfoCLEAR.vi"("Session info In"=w264) -> ("Session info Out"=w265:T12)  [unwired: 10 in]
                    n217 = local write "Session info"(w265) -> ()
                  }
                }
                n218 = case shown="True" w231 {
                  tunnel: w234 -> [w248 w255]
                  tunnel: [w249 w254] -> w233
                  tunnel: w229 -> [_ w253]
                  tunnel: w228 -> [w247 w252]
                  frame False {
                    n219 = call "pp3_trial_NextState.vi"("Reward CR"=w247, "New state countdown (ms)"=i64 0, "New State"=pp3_CTL_State."2 (Load Trial)", "State In"=w248) -> ("State Out"=w249:T9)  [unwired: 7 in]
                  }
                  frame True {
                    # "Habituation only if 0th trial and habituation length >0"
                    n220 = To Quad Integer(1:w253) -> (0:w256:i64)
                    n221 = Multiply(x=w256, y=i64 1000) -> (x*y=w257:i64)
                    n222 = call "pp3_trial_NextState.vi"("Reward CR"=w252, "New state countdown (ms)"=w257, "New State"=pp3_CTL_State."1 Habituation", "State In"=w255) -> ("State Out"=w254:T9)  [unwired: 7 in]
                  }
                }
                n223 = local write "State info"(w233) -> ()
              }
              frame #2 {
                w288 = "\t"
                # "Serialize DAQ configurations for logging que"
                # "Initialize logging queues and log directory"
                n224 = Get Date/Time In Seconds() -> (seconds since 1Jan1904=w305:timestamp)
                n225 = local read "Session parameters"() -> (w317:T11)
                n226 = Obtain Queue(name (unnamed)="RL Log Queue", element data type="") -> (queue out=w272:refnum<queue>)  [unwired: 3 in, 2 out]
                n227 = Unbundle By Name(w317) -> ("Log File Directory Root"=w304:path, "Subject Name"=w315:string)
                n228 = Format Date/Time String(time format string (%c)="\\%y%m%d\\%H%M%S\\", seconds (now)=w305) -> (date/time string=w316:string)  [unwired: 1 in]
                n229 = Format Date/Time String(time format string (%c)="%y%m%d_%H%M%S.pp2tt.tsv" ("pattern (all files)"), seconds (now)=w305) -> (date/time string=w313:string)  [unwired: 1 in]
                n230 = Format Date/Time String(time format string (%c)="%y%m%d_%H%M%S.pp2sl.tsv" ("pattern (all files)"), seconds (now)=w305) -> (date/time string=w307:string)  [unwired: 1 in]
                n231 = Format Date/Time String(time format string (%c)="%y%m%d_%H%M%S.pp2rl.tsv" ("pattern (all files)"), seconds (now)=w305) -> (date/time string=w303:string)  [unwired: 1 in]
                n232 = Open VI Reference(type specifier VI Refnum (for type only)=refnum<vi> refnum, vi path=path "C:/Packages/pyonpyon/LV2/impl/pp2_log_SpawnRLLogger.vi", options=128) -> (vi reference=w277:refnum<vi>, error out=w276:errorcluster)  [unwired: 3 in]
                n233 = Concatenate Strings(w315, w316) -> (w314:string)
                n234 = Build Path(base path=w304, name or relative path=w314) -> (appended path=w296:path)
                n235 = Create Folder(path (use dialog)=w296) -> (created path=w290:path)  [unwired: 2 in, 2 out]
                n236 = disable-structure shown="Disabled" {
                  disable-tunnel: w313 -> [w321 _]
                  disable-tunnel: w290 -> [w318 _]
                  frame Disabled {
                    (unwired) TRUE ("Actually Run?")
                    n237 = Build Path(base path=w318, name or relative path=w321) -> (appended path=w320:path)
                    n238 = local read "Trial Types"() -> (w319:T1[])
                    n239 = call "pp3_log_trialTypes.vi"("Trial Types File Path"=w320, "Trial Types"=w319) -> ()  [unwired: 10 in]
                  }
                  frame Enabled {
                  }
                }
                n240 = Build Path(base path=w290, name or relative path=w303) -> (appended path=w273:path)
                n241 = call-by-ref "Start Asynchronous Call"(reference=w277, error in=w276, "file path in"=w273, "queue in"=w272) -> ()  [unwired: 10 in, 2 out]
                n242 = Build Path(base path=w290, name or relative path=w307) -> (appended path=w298:path)
                n243 = local read "Session List Hidden"() -> (w309:u8[])
                n244 = Bundle By Name(cluster=w317, "Log File Directory"=w290) -> (w270:T11)
                n245 = local read "Daq config"() -> (w312:T4)
                n246 = Build Path(base path=w290, name or relative path="cam\\") -> (appended path=w294:path)
                n247 = local read "Info Hostname"() -> (w287:string)
                n248 = local read "Info VI Revision"() -> (w286:string)
                n249 = Create Folder(path (use dialog)=w294) -> ()  [unwired: 2 in, 3 out]
                n250 = call "pp3b_log_DAQconfig.vi"("queue in"=w272, "Daq config"=w312) -> ("queue out"=w284:refnum<queue>)  [unwired: 9 in]
                n251 = call "pp2_log_toString_sessionList.vi"("Session List in"=w309) -> ("spreadsheet string"=w308:string)  [unwired: 10 in]
                n252 = local write "Session parameters"(w270) -> ()
                n253 = call "pp3_log_sessionParameters.vi"("queue in"=w284) -> ("queue out"=w292:refnum<queue>)  [unwired: 10 in]
                n254 = Open/Create/Replace File(file path (use dialog)=w298, operation (0:open)=T14."create") -> (refnum out=w299:refnum<file>)  [unwired: 4 in, 2 out]
                n255 = call "pp3_log_trialMemo.vi"("queue in"=w292) -> ("queue out"=w293:refnum<queue>)  [unwired: 10 in]
                n256 = Concatenate Strings("RUNLOG" ("string"), w288, w287, w288, " " ("string"), w288, w286, "\r") -> (w282:string)
                n257 = call "pp3_log_state.vi"("Log memo?"=TRUE, "queue in"=w293) -> ("queue out"=w283:refnum<queue>)  [unwired: 9 in]
                n258 = Write to Text File(file (use dialog)=w299, text=w308) -> (refnum out=w310:refnum<file>, error out=w311:errorcluster)  [unwired: 2 in, 1 out]
                n259 = Close File(refnum=w310, error in=w311) -> ()  [unwired: 2 out]
                n260 = Enqueue Element(queue=w283, element=w282) -> (queue out=w281:refnum<queue>)  [unwired: 2 in, 2 out]
              }
              frame #3 {
                w333 = 1000 ("y")
                # "Stop whole VI if \"Stop\" pushed or end reached"
                # "Main Behavior Loop"
                n261 = local read "Session parameters"() -> (w352:T11)
                n262 = Unbundle By Name(w352) -> ("ITI max\n(s)"=w340:i32, "ITI min\n(s)"=w339:i32, "Stay \n(s)"=w353:i32, "Jump time\n(s)"=w348:i32, "Shock \ndur (s)"=w347:i32, "Pre click \n(V)"=w344:dbl, "Click\ndel (s)"=w332:dbl, "Reward CR"=w323:bool)
                n263 = local read "Session info"() -> (w327:T12)
                n264 = local read "Runtime Errors"() -> (w335:errorcluster)
                n265 = local read "Daq config"() -> (w334:T4)
                n266 = local read "State info"() -> (w328:T9)
                n267 = Multiply(x=w333, y=w340) -> (x*y=w342:i32)
                n268 = Multiply(x=w333, y=w339) -> (x*y=w341:i32)
                n269 = Multiply(x=w353, y=w333) -> (x*y=w354:i32)
                n270 = Multiply(x=w348, y=w333) -> (x*y=w350:i32)
                n271 = Multiply(x=w347, y=w333) -> (x*y=w349:i32)
                n272 = Multiply(x=w332, y=w333) -> (x*y=w331:dbl)
                n273 = To Quad Integer(1:w341) -> (0:w337:i64)
                n274 = To Quad Integer(1:w350) -> (0:w346:i64)
                n275 = To Quad Integer(1:w342) -> (0:w338:i64)
                n276 = To Quad Integer(1:w354) -> (0:w351:i64)
                n277 = To Quad Integer(1:w349) -> (0:w345:i64)
                n278 = To Quad Integer(1:w331) -> (0:w330:i64)
                n279 = while {
                  shift-right: [w385] -> w329
                  shift-left: w328 -> [w384]
                  shift-right: [w383] -> _
                  shift-left: w327 -> [w388]
                  shift-right: [w367] -> w324
                  shift-left: w326 -> [w361]
                  tunnel: w351 -> [w382]
                  tunnel: w346 -> [w381]
                  tunnel: w345 -> [w380]
                  tunnel: w344 -> [w379]
                  shift-right: [w378] -> w336
                  shift-left: w335 -> [w371]
                  shift-right: [w376] -> _
                  shift-left: FALSE -> [w377]
                  tunnel: w338 -> [w375]
                  tunnel: w337 -> [w374]
                  tunnel: w330 -> [w368]
                  tunnel: [w364] -> w325
                  tunnel: w323 -> [w358]
                  shift-right: [w357] -> w322
                  shift-left: w334 -> [w356]
                  stop <- w370 stop-if-true
                  # "Update error display here"
                  # "Pre click (V)"
                  # "Click del (ms)"
                  # "Jump time (ms)"
                  # "Stay (ms)"
                  # "ITI max/min (ms)"
                  # "Shock dur (ms)"
                  # "Done and timed out"
                  # "Exitable?"
                  # "Once marker\n(reset to False automatically\nat loop end for most types)"
                  # "State timeout?"
                  # "Side changed?"
                  n280 = call "pp3_updateSideState.vi"("error in (no error)"=w371, "log queue in"=w361, "Daq config In"=w356, "State In"=w384) -> ("error out"=w372:errorcluster, "log queue out"=w360:refnum<queue>, "State Out"=w359:T9, "State timeout"=w387:bool, "Side change"=w386:bool)  [unwired: 2 in, 1 out]
                  n281 = local write "Runtime Errors"(w371) -> ()
                  n282 = case shown="True" TRUE {
                    tunnel: w359 -> [_ w389]
                    frame False {
                    }
                    frame True {
                      n283 = local write "State info"(w389) -> ()
                    }
                  }
                  n284 = Unbundle By Name(w359) -> ("Curr State"=w369:T10)
                  n285 = case shown="\"0 NULL\", \"15 Done\"" w369 {
                    selector: w369 -> [_ _ _ _ w518 _ _ _ _]
                    tunnel: w388 -> [w399 w421 w439 w488 w524 w588 w619 w639 w691]
                    tunnel: w359 -> [w401 w413 w443 w479 w528 w592 w623 w640 w690]
                    tunnel: w387 -> [w393 _ w440 w486 w526 w591 _ w644 w688]
                    tunnel: w386 -> [_ _ w444 _ w529 w590 _ _ _]
                    tunnel: [w400 w425 w442 w489 w527 w595 w622 w643 w690] -> w385
                    tunnel: [w399 w421 w439 w488 w524 w588 w619 w638 w691] -> w383
                    tunnel: w382 -> [_ w422 w441 _ _ _ _ _ _]
                    tunnel: w381 -> [_ _ _ w490 _ _ _ _ _]
                    tunnel: w380 -> [_ _ _ _ w525 _ _ _ _]
                    tunnel: w379 -> [_ _ w434 _ _ _ _ _ _]
                    tunnel: w372 -> [w397 w420 w438 w482 w522 w584 w618 w635 w692]
                    tunnel: [w397 w419 w437 w481 w521 w583 w618 w634 w692] -> w378
                    tunnel: w377 -> [_ _ _ w484 _ _ _ w642 w693]
                    tunnel: [FALSE FALSE FALSE w483 FALSE FALSE FALSE w641 w693] -> w376
                    tunnel: w375 -> [_ _ _ _ _ w594 w625 _ _]
                    tunnel: w374 -> [_ _ _ _ _ w593 w624 _ _]
                    tunnel: [TRUE FALSE FALSE FALSE FALSE FALSE FALSE TRUE TRUE] -> w373
                    tunnel: w368 -> [_ _ w433 _ _ _ _ _ _]
                    tunnel: w360 -> [w394 w411 w432 w485 w519 w586 w616 w636 w689]
                    tunnel: [w394 w410 w432 w485 w519 w586 w616 w636 w689] -> w367
                    tunnel: [FALSE ("State timeout") FALSE ("State timeout") FALSE ("State timeout") FALSE ("State timeout") FALSE ("State timeout") FALSE ("State timeout") FALSE ("State timeout") FALSE ("State timeout") w688] -> w362
                    tunnel: w358 -> [w391 w409 w429 w476 w515 w582 w614 w630 _]
                    tunnel: [w390 w408 w428 w475 w513 w581 w613 w628 w686] -> w357
                    tunnel: w356 -> [w390 w408 w427 w474 w514 w580 w613 w629 w686]
                    frame "1 Habituation" {
                      n286 = case shown="True" w393 {
                        tunnel: w401 -> [w402 w407]
                        tunnel: [w402 w406] -> w400
                        tunnel: w391 -> [_ w403]
                        frame False {
                        }
                        frame True {
                          # "Load next if timeout"
                          n287 = call "pp3_trial_NextState.vi"("Reward CR"=w403, "New state countdown (ms)"=i64 0, "New State"=pp3_CTL_State."2 (Load Trial)", "State In"=w407) -> ("State Out"=w406:T9)  [unwired: 7 in]
                        }
                      }
                      n288 = Wait Until Next ms Multiple(millisecond multiple=u32 3) -> ()  [unwired: 1 out]
                    }
                    frame "2 (Load Trial)" {
                      # "Load curr trial and apply variable shock if on.\n(will not increment)"
                      n289 = local read "Session param (dynamic)"() -> (w416:T8)
                      n290 = local read "Session List Hidden"() -> (w417:u8[])
                      n291 = disable-structure shown="Disabled" {
                        frame Disabled {
                          n292 = Wait Until Next ms Multiple(millisecond multiple=u32 1) -> ()  [unwired: 1 out]
                        }
                        frame Enabled {
                        }
                      }
                      n293 = local read "Trial Types"() -> (w418:T1[])
                      n294 = call "pp3_trial_loadNext.vi"("State Info In"=w413, "Session param (dynamic)"=w416, "Session List (Hidden variable)"=w417, "Trial Types"=w418, "Daq config In"=w408, "log queue in"=w411, "error in (no error)"=w420) -> ("State Info Out"=w424:T9, "log queue out"=w410:refnum<queue>, "error out"=w419:errorcluster)  [unwired: 6 in]
                      n295 = call "pp3_trial_NextState.vi"("Reward CR"=w409, "New state countdown (ms)"=w422, "New State"=pp3_CTL_State."3 Stay Period", "State In"=w424) -> ("State Out"=w425:T9)  [unwired: 7 in]
                    }
                    frame "3 Stay Period" {
                      n296 = case shown="False" w444 {
                        tunnel: w443 -> [w454 w473]
                        tunnel: [w449 w472] -> w442
                        tunnel: w441 -> [_ w470]
                        tunnel: w440 -> [w453 _]
                        tunnel: w438 -> [w452 w469]
                        tunnel: [w451 w469] -> w437
                        tunnel: [w450 w467] -> w428
                        tunnel: w434 -> [w448 _]
                        tunnel: w433 -> [w447 _]
                        tunnel: w429 -> [w446 w468]
                        tunnel: w427 -> [w445 w467]
                        frame False {
                          n297 = case shown="True" w453 {
                            tunnel: w454 -> [w457 w466]
                            tunnel: w452 -> [w456 w464]
                            tunnel: [w456 w463] -> w451
                            tunnel: [w455 w458] -> w450
                            tunnel: [w457 w462] -> w449
                            tunnel: w448 -> [_ w461]
                            tunnel: w447 -> [_ w460]
                            tunnel: w446 -> [_ w459]
                            tunnel: w445 -> [w455 w458]
                            frame False {
                              # "No side change, no timeout"
                            }
                            frame True {
                              # "If stay timed out without side change, \ntrigger change to (Load audio) and play click"
                              n298 = call "pp3_trial_NextState.vi"("Reward CR"=w459, "New state countdown (ms)"=w460, "New State"=pp3_CTL_State."4 Load Audio/Click Delay", "State In"=w466) -> ("State Out"=w462:T9)  [unwired: 7 in]
                              n299 = call "pp3_DAQ_AudioClick.vi"("State In"=w462, "Daq config"=w458, "Pre click \n(V)"=w461, "error in (no error)"=w464) -> ("error out"=w463:errorcluster)  [unwired: 6 in]
                            }
                          }
                        }
                        frame True {
                          # "If side changed during stay, reload stay period\n(will not log state change, 3 == 3)"
                          n300 = call "pp3_trial_NextState.vi"("Reward CR"=w468, "New state countdown (ms)"=w470, "New State"=pp3_CTL_State."3 Stay Period", "State In"=w473) -> ("State Out"=w472:T9)  [unwired: 7 in]
                        }
                      }
                      n301 = Wait Until Next ms Multiple(millisecond multiple=u32 1) -> ()  [unwired: 1 out]
                    }
                    frame "4 Load Audio/Click Delay" {
                      n302 = case shown="False" w484 {
                        selector: w484 -> [_ w501]
                        tunnel: [TRUE w501] -> w483
                        tunnel: w482 -> [w497 w502]
                        tunnel: [w496 w499] -> w475
                        tunnel: [w495 w502] -> w481
                        tunnel: w479 -> [w494 w500]
                        tunnel: [w492 w500] -> w478
                        tunnel: w474 -> [w491 w499]
                        frame False {
                          # "Load audio just once"
                          n303 = call "pp3_DAQ_AudioLoadStimulus.vi"("State Info In"=w494, "Daq config In"=w491, "error in (no error)"=w497) -> ("Daq config Out"=w496:T4, "error out"=w495:errorcluster)  [unwired: 11 in]
                          n304 = Bundle By Name(cluster=w494, "Tone countdown (ms)"=i64 0) -> (w492:T9)
                        }
                        frame True {
                        }
                      }
                      n305 = case shown="True" w486 {
                        tunnel: w490 -> [_ w507]
                        tunnel: [w503 w508] -> w489
                        tunnel: w478 -> [w503 w505]
                        tunnel: w476 -> [_ w504]
                        frame False {
                        }
                        frame True {
                          n306 = Unbundle By Name(w505) -> ("Current Loaded Trial.Trial Type"=w509:T2)
                          n307 = case shown="\"TEST\", Default" w509 {
                            tunnel: [pp3_CTL_State."5 GO Trial" ("New State") pp3_CTL_State."11 TEST Trial" ("New State") pp3_CTL_State."8 NOGO Trial" ("New State")] -> w506
                            frame "GO" {
                            }
                            frame "TEST", Default {
                            }
                            frame "NOGO" {
                            }
                          }
                          n308 = call "pp3_trial_NextState.vi"("Reward CR"=w504, "New state countdown (ms)"=w507, "New State"=w506, "State In"=w505) -> ("State Out"=w508:T9)  [unwired: 7 in]
                        }
                      }
                      n309 = Wait Until Next ms Multiple(millisecond multiple=u32 1) -> ()  [unwired: 1 out]
                    }
                    frame "5 GO Trial", "8 NOGO Trial", "11 TEST Trial" {
                      n310 = case shown="False" w529 {
                        tunnel: w528 -> [w538 w569]
                        tunnel: [w537 w571] -> w527
                        tunnel: w526 -> [w539 _]
                        tunnel: w525 -> [w536 w565]
                        tunnel: [w535 w563] -> w513
                        tunnel: w522 -> [w534 w570]
                        tunnel: [w533 w570] -> w521
                        tunnel: w518 -> [w532 w568]
                        tunnel: w515 -> [w531 w564]
                        tunnel: w514 -> [w530 w563]
                        frame False {
                          n311 = case shown="False" w539 {
                            tunnel: w538 -> [w542 w554]
                            tunnel: [w541 w553] -> w537
                            tunnel: w536 -> [_ w549]
                            tunnel: [w545 w546] -> w535
                            tunnel: w534 -> [w544 w552]
                            tunnel: [w543 w552] -> w533
                            tunnel: w532 -> [_ w548]
                            tunnel: w531 -> [_ w547]
                            tunnel: w530 -> [w540 w546]
                            frame False {
                              # "continue/start  sound,\nretrigger if necessary"
                              n312 = call "pp3_DAQ_AudioTriggerPlay.vi"("Daq config In"=w540, "State In"=w542, "error in (no error)"=w544) -> ("Daq config Out"=w545:T4, "State Out"=w541:T9, "error out"=w543:errorcluster)  [unwired: 10 in]
                            }
                            frame True {
                              n313 = case shown="Default" w548 {
                                selector: w548 -> [w556 _ _ _]
                                tunnel: [w556 pp3_CTL_State."7 GO Timeout" ("New State") pp3_CTL_State."10 NOGO Timeout" ("New State") pp3_CTL_State."13 TEST Timeout" ("New State")] -> w551
                                tunnel: [i64 0 ("New state countdown (ms)") w557 i64 0 ("New state countdown (ms)") i64 0 ("New state countdown (ms)")] -> w550
                                tunnel: w549 -> [_ w557 _ _]
                                frame Default {
                                # "Will not happen"
                                }
                                frame "5 GO Trial" {
                                # "If timout, miss!!!"
                                }
                                frame "8 NOGO Trial" {
                                # "If time out,\ncorrect rejection!!!"
                                }
                                frame "11 TEST Trial" {
                                }
                              }
                              n314 = call "pp3_trial_NextState.vi"("Reward CR"=w547, "New state countdown (ms)"=w550, "New State"=w551, "State In"=w554) -> ("State Out"=w553:T9)  [unwired: 7 in]
                            }
                          }
                        }
                        frame True {
                          n315 = case shown="\"5 GO Trial\"" w568 {
                            selector: w568 -> [w573 _ _ _]
                            tunnel: [w573 pp3_CTL_State."6 GO Jumped" ("New State") pp3_CTL_State."9 NOGO Jumped" ("New State") pp3_CTL_State."12 TEST Jumped" ("New State")] -> w566
                            tunnel: [i64 0 ("New state countdown (ms)") i64 0 ("New state countdown (ms)") w576 i64 0 ("New state countdown (ms)")] -> w567
                            tunnel: w565 -> [_ _ w576 _]
                            frame Default {
                              # "Will not happen"
                            }
                            frame "5 GO Trial" {
                              # "If side changed, hit!!!"
                            }
                            frame "8 NOGO Trial" {
                              # "If side changed,\nfalse alarm!!!"
                            }
                            frame "11 TEST Trial" {
                              # "If side changed, hit!!!"
                            }
                          }
                          n316 = call "pp3_trial_NextState.vi"("Reward CR"=w564, "New state countdown (ms)"=w567, "New State"=w566, "State In"=w569) -> ("State Out"=w571:T9)  [unwired: 7 in]
                        }
                      }
                      n317 = Wait Until Next ms Multiple(millisecond multiple=u32 1) -> ()  [unwired: 1 out]
                    }
                    frame "7 GO Timeout", "9 NOGO Jumped" {
                      # "Shock end should be ASAP"
                      n318 = Or(x=w590, y=w591) -> (x .or. y?=w589:bool)
                      n319 = case shown="False" w589 {
                        tunnel: [w599 w611] -> w595
                        tunnel: w594 -> [_ w610]
                        tunnel: w593 -> [_ w609]
                        tunnel: w592 -> [w600 w607]
                        tunnel: [w603 w604] -> w581
                        tunnel: w584 -> [w602 w606]
                        tunnel: [w601 w606] -> w583
                        tunnel: w582 -> [_ w605]
                        tunnel: w580 -> [w598 w604]
                        frame False {
                          # "continue/start  sound,\nretrigger if necessary"
                          # "Continue shock"
                          n320 = call "pp3_DAQ_AudioTriggerPlay.vi"("Daq config In"=w598, "State In"=w600, "error in (no error)"=w602) -> ("Daq config Out"=w603:T4, "State Out"=w599:T9, "error out"=w601:errorcluster)  [unwired: 10 in]
                        }
                        frame True {
                          # "If side change or timeout,\nnext state (end shock)"
                          n321 = call "RandomInt64.vi"("Min"=w609, "Max"=w610) -> ("Random"=w608:i64)  [unwired: 9 in]
                          n322 = call "pp3_trial_NextState.vi"("Reward CR"=w605, "New state countdown (ms)"=w608, "New State"=pp3_CTL_State."14 Intertrial Interval", "State In"=w607) -> ("State Out"=w611:T9)  [unwired: 7 in]
                        }
                      }
                      n323 = disable-structure shown="Disabled" {
                        frame Disabled {
                          n324 = Wait Until Next ms Multiple(millisecond multiple=u32 1) -> ()  [unwired: 1 out]
                        }
                        frame Enabled {
                        }
                      }
                    }
                    frame "6 GO Jumped", "10 NOGO Timeout", "12 TEST Jumped", "13 TEST Timeout" {
                      # "Response correct,\ngo to ITI immediately"
                      n325 = disable-structure shown="Disabled" {
                        frame Disabled {
                          n326 = Wait Until Next ms Multiple(millisecond multiple=u32 1) -> ()  [unwired: 1 out]
                        }
                        frame Enabled {
                        }
                      }
                      n327 = call "RandomInt64.vi"("Min"=w624, "Max"=w625) -> ("Random"=w621:i64)  [unwired: 9 in]
                      n328 = call "pp3_trial_NextState.vi"("Reward CR"=w614, "New state countdown (ms)"=w621, "New State"=pp3_CTL_State."14 Intertrial Interval", "State In"=w623) -> ("State Out"=w622:T9)  [unwired: 7 in]
                    }
                    frame "14 Intertrial Interval" {
                      n329 = case shown="False" w642 {
                        selector: w642 -> [_ w670]
                        tunnel: [TRUE w670] -> w641
                        tunnel: w640 -> [w649 w667]
                        tunnel: w639 -> [w659 w669]
                        tunnel: [w656 w669] -> w638
                        tunnel: w635 -> [w654 w668]
                        tunnel: [w657 w668] -> w634
                        tunnel: [w658 w666] -> w628
                        tunnel: [w655 w667] -> w631
                        tunnel: w629 -> [w645 w666]
                        frame False {
                          # "Paint done trial in table"
                          # "Runs just first cycle!"
                          # "Update stats/close audio"
                          n330 = call "pp3_updateSessionInfo.vi"("Session info In"=w659, "State In"=w649) -> ("Session info Out"=w656:T12)  [unwired: 9 in]
                          n331 = Unbundle By Name(w649) -> ("Curr  tr"=w647:u16, "Prev State"=w650:T10)
                          n332 = local write "Session info"(w656) -> ()
                          n333 = call "pp3_DAQ_AudioWaitStop.vi"("State info"=w649, "Daq config In"=w645, "error in (no error)"=w654) -> ("State info out"=w651:T9, "Daq config Out"=w658:T4, "error out"=w657:errorcluster)  [unwired: 10 in]
                          n334 = case shown="\"9 NOGO Jumped\"" w650 {
                            tunnel: [u32 52736 u32 11206570 u32 16731983 u32 16763594 u32 12369084] -> w648
                            frame "6 GO Jumped" {
                            }
                            frame "7 GO Timeout" {
                            }
                            frame "9 NOGO Jumped" {
                            }
                            frame "10 NOGO Timeout" {
                            }
                            frame Default {
                            }
                          }
                          n335 = Bundle By Name(cluster=w651, "Tone\nGate"=FALSE ("Tone\nGate"), "State update flag"=TRUE) -> (w655:T9)
                          n336 = control-ref of="Session list display"() -> (w646:refnum<vi>)
                          n337 = call "pp2_util_paintTableElement.vi"("Color Box"=w648, "Numeric"=w647, "Tbl Refnum"=w646) -> ()  [unwired: 9 in]
                        }
                        frame True {
                        }
                      }
                      n338 = Wait Until Next ms Multiple(millisecond multiple=u32 3) -> ()  [unwired: 1 out]
                      n339 = case shown="True" w644 {
                        tunnel: [w671 w679] -> w643
                        tunnel: w631 -> [w671 w673]
                        tunnel: w630 -> [_ w672]
                        frame False {
                        }
                        frame True {
                          # "Exit if last trial fin\n15s extra video"
                          n340 = Unbundle By Name(w673) -> ("Curr  tr"=w681:u16, "Total trials memo"=w677:i64)
                          n341 = Increment(x=w681) -> (x+1=w675:u16)
                          n342 = Greater Or Equal?(x=w675, y=w677) -> (x >= y?=w676:bool)
                          n343 = case shown="False" w676 {
                            tunnel: [pp3_CTL_State."15 Done" ("New State") pp3_CTL_State."2 (Load Trial)" ("New State")] -> w678
                            tunnel: [i64 15000 ("New state countdown (ms)") i64 0 ("New state countdown (ms)")] -> w674
                            frame True {
                            }
                            frame False {
                            }
                          }
                          n344 = Bundle By Name(cluster=w673, "Curr  tr"=w675) -> (w680:T9)
                          n345 = call "pp3_trial_NextState.vi"("Reward CR"=w672, "New state countdown (ms)"=w674, "New State"=w678, "State In"=w680) -> ("State Out"=w679:T9)  [unwired: 7 in]
                        }
                      }
                    }
                    frame "0 NULL", "15 Done" {
                      # "When \"15 Done\" times out,\nsignal will be sent to exit the \nloop"
                      # "\"0 Null\" Will not happen, added to fix compile error"
                      n346 = Wait Until Next ms Multiple(millisecond multiple=u32 3) -> ()  [unwired: 1 out]
                    }
                  }
                  n347 = local read "stop"() -> (w366:bool)
                  n348 = Or(x=w366, y=w362) -> (x .or. y?=w364:bool)
                  n349 = Or(x="Pause", y=w364) -> (x .or. y?=w363:bool)
                  n350 = And(x=w373, y=w363) -> (x .and. y?=w370:bool)
                }
                n351 = local write "State info"(w329) -> ()
                n352 = local write "Daq config"(w322) -> ()
              }
              frame #4 {
                # "Will close log file"
                n353 = flat-sequence {
                  frame #0 {
                    # "This done in \"15 Done\"\nloop instead"
                    n354 = disable-structure shown="Disabled" {
                      frame Disabled {
                        # "Always record at least\n10 extra seconds of video"
                        n355 = Wait (ms)(milliseconds to wait=u32 10000) -> ()  [unwired: 1 out]
                      }
                      frame Enabled {
                      }
                    }
                  }
                  frame #1 {
                    w700 = FALSE
                    # "This will stop webcam recording in\nasynchronous processs"
                    n356 = local read "State info"() -> (w701:T9)
                    n357 = Bundle By Name(cluster=w701, "Tone\nGate"=w700, "Punish"=w700, "Current DAQ DO Int"=u16 0, "Webcam recording"=w700) -> (w702:T9)
                    n358 = local write "State info"(w702) -> ()
                  }
                }
                n359 = Release Queue(queue=w695, error in (no error)=w696) -> (error out=w697:errorcluster)  [unwired: 1 in, 2 out]
                n360 = local write "Runtime Errors"(w697) -> ()
              }
              frame #5 {
                # "Post-behavior UI adjustments"
                n361 = local read "Runtime Errors"() -> (w704:errorcluster)
                n362 = local read "Daq config"() -> (w706:T4)
                n363 = property on="Pause" class="Bool (strict)"("DisabledEnum"=T13."Disabled and Grayed Out" ("Disabled")) -> ()  [unwired: 2 in, 2 out]
                n364 = property on="Trial Types Control" class="TabCtl (strict)"("DisabledEnum"=T13."Enabled" ("Disabled")) -> ()  [unwired: 2 in, 2 out]
                n365 = call "pp3b_DAQwriteDO.vi"("error in (no error)"=w704, "Daq config"=w706, "DAQ Digital In"=u16 0) -> ("error out"=w703:errorcluster)  [unwired: 8 in]
                n366 = local write "Runtime Errors"(w703) -> ()
              }
            }
          }
          event "60 trials": Value Change {
            n367 = event-data() -> ()  [unwired: 1 in, 6 out]
            n368 = local read "Session parameters"() -> (w715:T11)
            n369 = Bundle By Name(cluster=w715, "Habit tr0 (s)"=180, "ITI min\n(s)"=14 ("ITI min\n(s)"), "ITI max\n(s)"=24 ("ITI max\n(s)"), "Stay \n(s)"=5 ("Stay \n(s)")) -> (w714:T11)
            n370 = local write "Session parameters"(w714) -> ()
          }
          event "90 trials": Value Change {
            n371 = event-data() -> ()  [unwired: 1 in, 6 out]
            n372 = local read "Session parameters"() -> (w722:T11)
            n373 = Bundle By Name(cluster=w722, "Habit tr0 (s)"=180, "ITI min\n(s)"=6 ("ITI min\n(s)"), "ITI max\n(s)"=16 ("ITI max\n(s)"), "Stay \n(s)"=3 ("Stay \n(s)")) -> (w721:T11)
            n374 = local write "Session parameters"(w721) -> ()
          }
          event "test trials": Value Change {
            n375 = event-data() -> ()  [unwired: 1 in, 6 out]
            n376 = local read "Session parameters"() -> (w729:T11)
            n377 = Bundle By Name(cluster=w729, "Habit tr0 (s)"=5, "ITI min\n(s)"=5 ("ITI min\n(s)"), "ITI max\n(s)"=5 ("ITI max\n(s)"), "Stay \n(s)"=3 ("Stay \n(s)")) -> (w728:T11)
            n378 = local write "Session parameters"(w728) -> ()
          }
        }
      }
    }
    frame #4 {
      w739 = FALSE ("Webcam on")
      w742 = FALSE
      w738 = T13."Enabled" ("Disabled")
      # "Close task only if video used"
      # "Clean up DAQ"
      # "Stop webcam recording"
      # "Post UI Adjustments"
      n379 = local read "State info"() -> (w740:T9)
      n380 = Bundle By Name(cluster=w740, "Webcam on"=w739, "Webcam recording"=w739) -> (w741:T9)
      n381 = local write "State info"(w741) -> ()
      n382 = property on="Daq config" class="Clust (strict)"("DisabledEnum"=w738) -> ()  [unwired: 2 in, 2 out]
      n383 = property on="Session List Control" class="TabCtl (strict)"("DisabledEnum"=w738) -> ()  [unwired: 2 in, 2 out]
      n384 = property on="Trial Types Control" class="TabCtl (strict)"("DisabledEnum"=w738) -> ()  [unwired: 2 in, 2 out]
      n385 = property on="Session param (dynamic)" class="Clust (strict)"("DisabledEnum"=w738) -> ()  [unwired: 2 in, 2 out]
      n386 = property on="State info" class="Clust (strict)"("DisabledEnum"=w738) -> ()  [unwired: 2 in, 2 out]
      n387 = property on="Session parameters" class="Clust (strict)"("DisabledEnum"=w738) -> ()  [unwired: 2 in, 2 out]
      n388 = property on="Session info" class="Clust (strict)"("DisabledEnum"=w738) -> ()  [unwired: 2 in, 2 out]
      n389 = property on="Session list display" class="Tbl (strict)"("Visible"=TRUE) -> ()  [unwired: 2 in, 2 out]
      n390 = local read "Runtime Errors"() -> (w735:errorcluster)
      n391 = local read "Daq config"() -> (w736:T4)
      n392 = local write "stop"(w742) -> ()
      n393 = local write "Pause"(w742) -> ()
      n394 = call "pp3_DAQclear.vi"("error in (no error)"=w735, "Daq config in"=w736) -> ("error out"=w732:errorcluster, "Daq config out"=w737:T4)  [unwired: 8 in]
      n395 = local write "Daq config"(w737) -> ()
      n396 = case shown="True" w731 {
        tunnel: w734 -> [_ w746]
        tunnel: [w743 w745] -> w733
        tunnel: w732 -> [w743 w744]
        frame False {
        }
        frame True {
          n397 = Close Reference(reference=w746, error in (no error)=w744) -> (error out=w745:errorcluster)
        }
      }
      n398 = local write "Runtime Errors"(w733) -> ()
    }
    frame #5 {
      # "Take screenshot for records"
      n399 = local read "Session parameters"() -> (w753:T11)
      n400 = Unbundle By Name(w753) -> ("Log File Directory"=w754:path)
      n401 = control-ref of="This VI"() -> (w750:refnum<vi>)
      n402 = Format Date/Time String(time format string (%c)="%y%m%d_%H%M%S.pp2ss.png" ("pattern (all files)")) -> (date/time string=w751:string)  [unwired: 2 in]
      n403 = Build Path(base path=w754, name or relative path=w751) -> (appended path=w747:path)
      n404 = invoke class="VI" method="FP.Get Image"(reference=w750, "image depth"=24 ("Image Depth")) -> ("image data"=w748:T15)  [unwired: 4 in, 5 out]
      n405 = call <vilib>:"Write PNG File.vi"("image data"=w748, "path to PNG file"=w747) -> ()  [unwired: 8 in, 2 out]
    }
  }
